vi "信号光谱9 -grating.vi"() -> ()   [LabVIEW 2018]
uses:
  <vilib>/Utility/NIReport.llb/Report Type.ctl
  <vilib>/Instr/_visa.llb/VISA Configure Serial Port (Instr).vi
  <vilib>/addons/_office/excel.llb/Excel Get Data ([str]).vi
  <vilib>/Utility/file.llb/Write Delimited Spreadsheet (DBL).vi
  <vilib>/Utility/NIReport.llb/NI_report.lvclass
  <vilib>/Analysis/NI_AALBase.lvlib
  <vilib>/Utility/NIReport.llb/NI_ReportGenerationCore.lvlib
  <vilib>/addons/_office/NI_ReportGenerationToolkit.lvlib
  <vilib>/Utility/NIReport.llb/Excel/NI_Excel.lvclass
panel:
  in  "C=w-w0":dbl=1800.0 format="%#_13g"
  in  "Target WL 2":dbl=552.444
  in  "判断角度上限":dbl=4.0 format="%#_13g"
  in  "判断角度下限":dbl=1.0 format="%#_13g"
  in  "角度倍乘系数":dbl=1.5
  out "Δw2>C":bool=TRUE
  out "Δw1>C":bool=TRUE
  out "θi":dbl
  in  "上升下降沿/s":dbl format="%.2p"
  in  "延时/s":dbl format="%.2p"
  in  "占空比/%":dbl=3.0 format="%.2p"
  in  "高电平/V":dbl=4.0 format="%.2p"
  in  "频率/Hz":dbl=6000.0 format="%.3p"
  in  "低电平/V":dbl min=0.0 max=5.0 format="%.2p"
  in  "Enable":bool
  in  "上升下降沿":i32(ring)=1 items=["上升沿", "下降沿"]
  in  "输出信号波形":u16(ring) items=["Pulse"]
  out "Output":bool
  in  "VISA 信号发生器":refnum<visa-resource-name>="USB0::0x1AB1::0x0641::DG4E192200870::INSTR"
  out "Output 2":bool
  in  "Enable 2":bool
  in  "上升下降沿/s 2":dbl format="%.2p"
  in  "延时/s 2":dbl format="%.2p"
  in  "占空比/% 2":dbl=3.0 format="%.2p"
  in  "高电平/V 2":dbl=0.002 format="%.2p"
  in  "频率/Hz 2":dbl=6000.0 format="%.3p"
  in  "低电平/V 2":dbl min=0.0 max=5.0 format="%.2p"
  in  "上升下降沿 2":i32(ring)=1 items=["上升沿", "下降沿"]
  in  "输出信号波形 2":u16(ring) items=["Pulse"]
  in  "终止测量":bool
  in  "测量次数":i32=1
  out "angle":dbl
  out "图片地址":string
  in  "开光时间/ms":u32=50
  out "最终存储路径 2":path
  out "照明光error out":errorcluster
  in  "照明光":bool
  in  "stop bits (10: 1 bit)":u16(ring)=10 items=["1.0"=10, "1.5"=15, "2.0"=20]
  in  "parity (0:none)":enum16{"None", "Odd", "Even", "Mark", "Space"}(ring)
  in  "data bits (8)":u16=8 min=5 max=8 step=1
  in  "baud rate":u32=9600 caption="baud rate (115200)" min=9600 max=115200
  in  "照明光VISA":refnum<visa-resource-name>="COM5"
  out "正在测量":bool
  out "最终存储路径":path
  in  "停止程序":bool
  out "configure error out":errorcluster
  in  "设置参数":bool
  out "output control error  4":errorcluster
  in  "低电平持续输出":bool
  out "output control error  5":errorcluster
  out "output control error":errorcluster
  in  "开始测量":bool
  in  "channel输出口":i32(ring) items=["Channel 1", "Channel 2"]
  out "output control error":errorcluster
  out "Spectrum":cluster{"Y":dbl[], "Y":dbl[]}[](graph)
  out "波长范围":dbl[](array[numeric])
  in  "?":enum32{"IHR 550", "CCD"}(tab)
  in  "Move To\nTarget Positions":bool
  out "Current UniqueID":string="Mono4"
  in  "Mono ID":string(combo)="Mono1"
  in  "Connect":bool
  out "Initialized JY":bool=TRUE
  in  "Force\nInitialization":bool
  in  "Target Grating":string(combo)="2"
  out "Current Description":string="1" caption="Description"
  out "Grating Index":i32=1
  out "Current Grating":dbl=1200.0
  out "Units":string="nm"
  out "Current WL":dbl=897.9988
  out "Exit Mirror\nPosition":i32(ring)=2 items=["EntranceMirror", "ExitMirror", "Front", "Side"]
  out "Entrance Mirror\nPosition":i32(ring)=2 items=["EntranceMirror", "ExitMirror", "Front", "Side"]
  out "Units 2":string="mm"
  out "Front Entrance":dbl
  in  "Target WL":dbl=517.603
  in  "Exit Mirror":u16(ring)=3 caption="Target Position Exit Mirror" items=["Front"=2, "Side"=3]
  in  "Entrance Mirror":u16(ring)=2 caption="Target Position\nEntrance Mirror" items=["Front"=2, "Side"=3]
  in  "Target\nFront Entrance":dbl=2.0
  in  "操作":bool
  in  "Commande tab":T1(tab)
  in  "Area Number to Display":i32
  in  "Reformat":bool
  in  "GAIN":u16(ring)=2 caption="Device Name" items=["High Light", "Best Dynamic Range", "High Sensitivity"]
  in  "ADC":u16(ring) caption="Device Name" items=["20 kHz       ", " 1 MHz       ", " 1 MHz Ultra "]
  in  "Number of Areas :":u16=1 min=1 step=1
  in  "Integration time (ms) :":i16=1000
  out "Uniques ID":u16(ring) items=["CCD1", "CCD2"]
  in  "Device Name":u16(ring) items=["Synapse CCD (Lateral)", "Synapse_IGA (Axial)"]
  in  "Signal type :":enum16{"TTL Rising Edge", "TTL Falling Edge"}(ring)=enum."TTL Falling Edge"
  in  "Trigger Type :":u16(ring) items=["On Start"=1, "Per Acquisition"=2]
  in  "trigSigTypeString":string
  in  "trigEventString":string
  in  "Enable InputTriggers :":bool
  in  "Number of Cleans":i32=1
  in  "MultiAcqShutterMode":i32(ring)=3 items=["Open For All Spectra"=1, "Open for Each Spectrum"=3]
  in  "Accumulations:":u16=10 min=1 step=1
  in  "Multi Accumulation mode:":bool
  out "Y Pixels:":i32=256
  out "DataSize":i32=1024
  out "X Pixels:":i32=1024
  out "Firmware\nVersion":string="V1.20 CCD_4000"
  out "initialized ?":bool=TRUE
  in  "Continuous":bool
  in  "CCD Busy":bool
  out "indicator":string="Ready !"
  in  "initialize":bool
  in  "ShutterOpen":bool=TRUE caption="Shutter enable"
  in  "Acquire":bool
  in  "Temperature":bool
  in  "Setup":bool
  out "Acq Time(ms)":u32=3401
  in  "Save Backlight":bool
  in  "cut backlight":bool
  out "backlight":bool=TRUE
  in  "是否保存":bool
  in  "Close":bool=TRUE
  out "JYCCDLib.IJYCCDReqd":refnum<k7>
  out "areas :":i32[][](array[numeric])=[[1], [1], [1], [1024], [256], [1], [256]]
  in  "Constante de condition\n(Voir l'aide contextuelle)":bool
  out "temp graph":dbl(graph)=-134.538067
  out "ADC Number":i32[](array[numeric])=[0, 1, 2, 3, 4]
  out "Gain Number":i32[](array[numeric])=[10, 11, 12, 13, 8, 2]
  out "trigAddress":i32
  out "Data":i32[][](graph)
  out "error out":errorcluster
  out "Gratings":dbl[](array[numeric])=[1200.0, 300.0]
  out "Backlight":i32[][](graph)
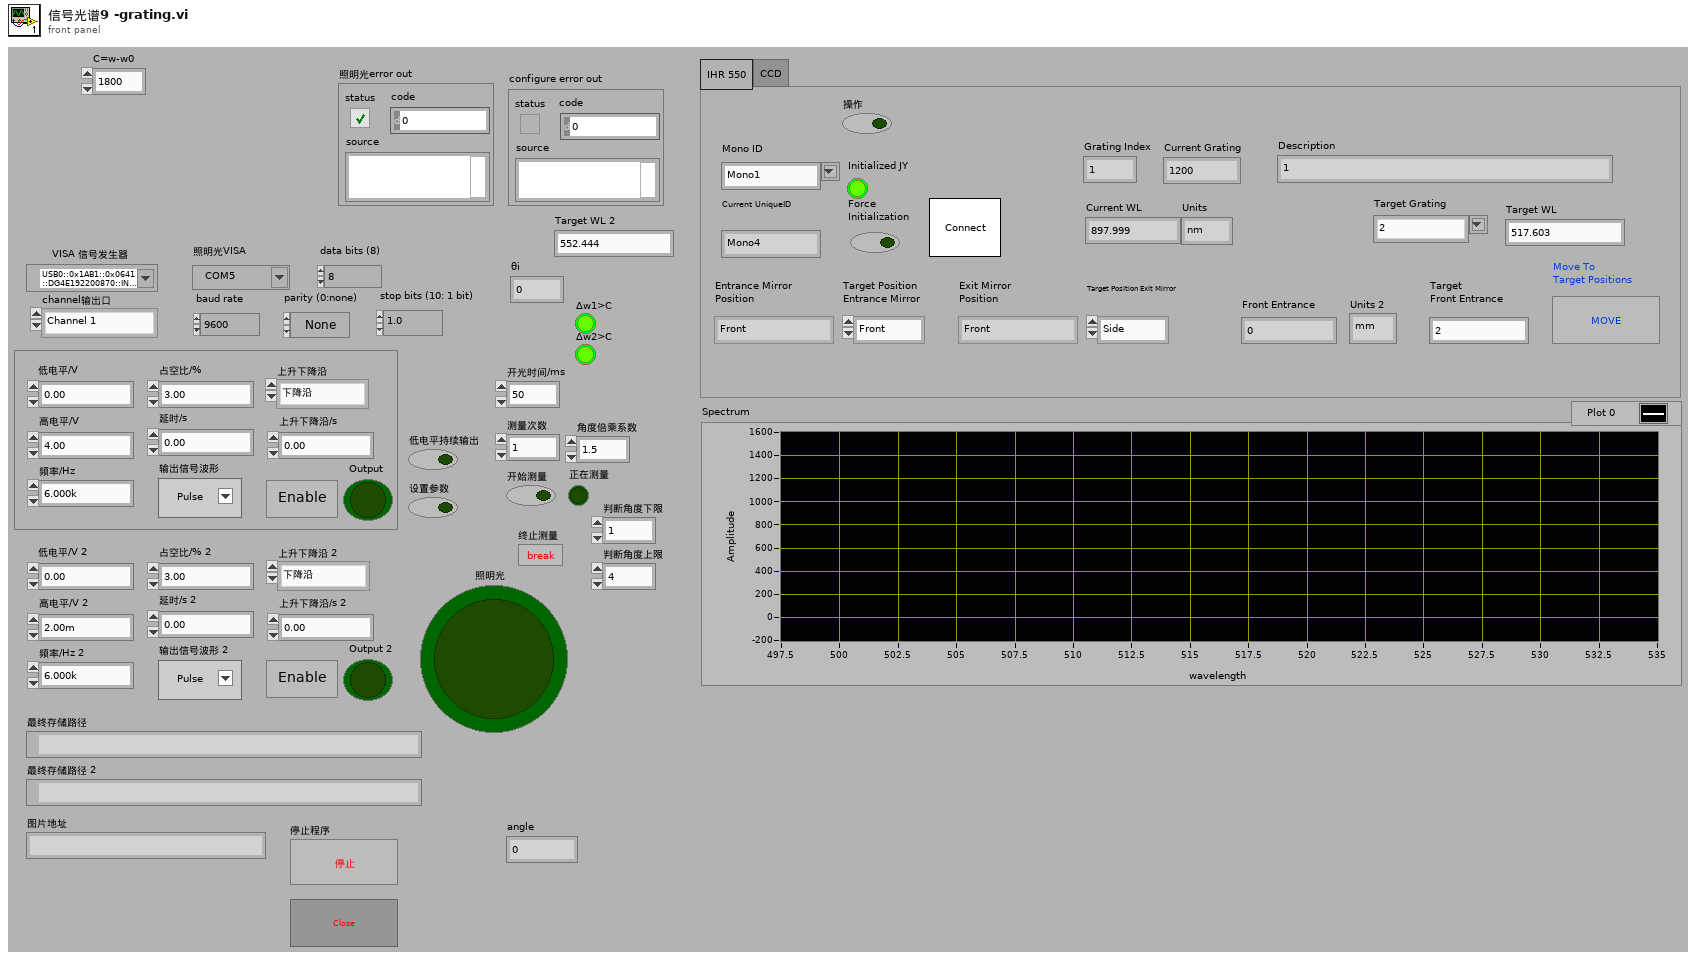
[diagram p1: front panel]
types:
  T1 = enum32{"Settings", "Trigger In", "Multi-Accu.", "Infos"}
  T2 = enum8{"Enabled", "Disabled", "Disabled and Grayed Out"}
  T3 = enum16{"maximized", "minimized", "normal", "no change"}
  T4 = typedef "NI_ReportGenerationCore.lvlib/Report Type.ctl" = enum16{"HTML", "Word", "Excel"}
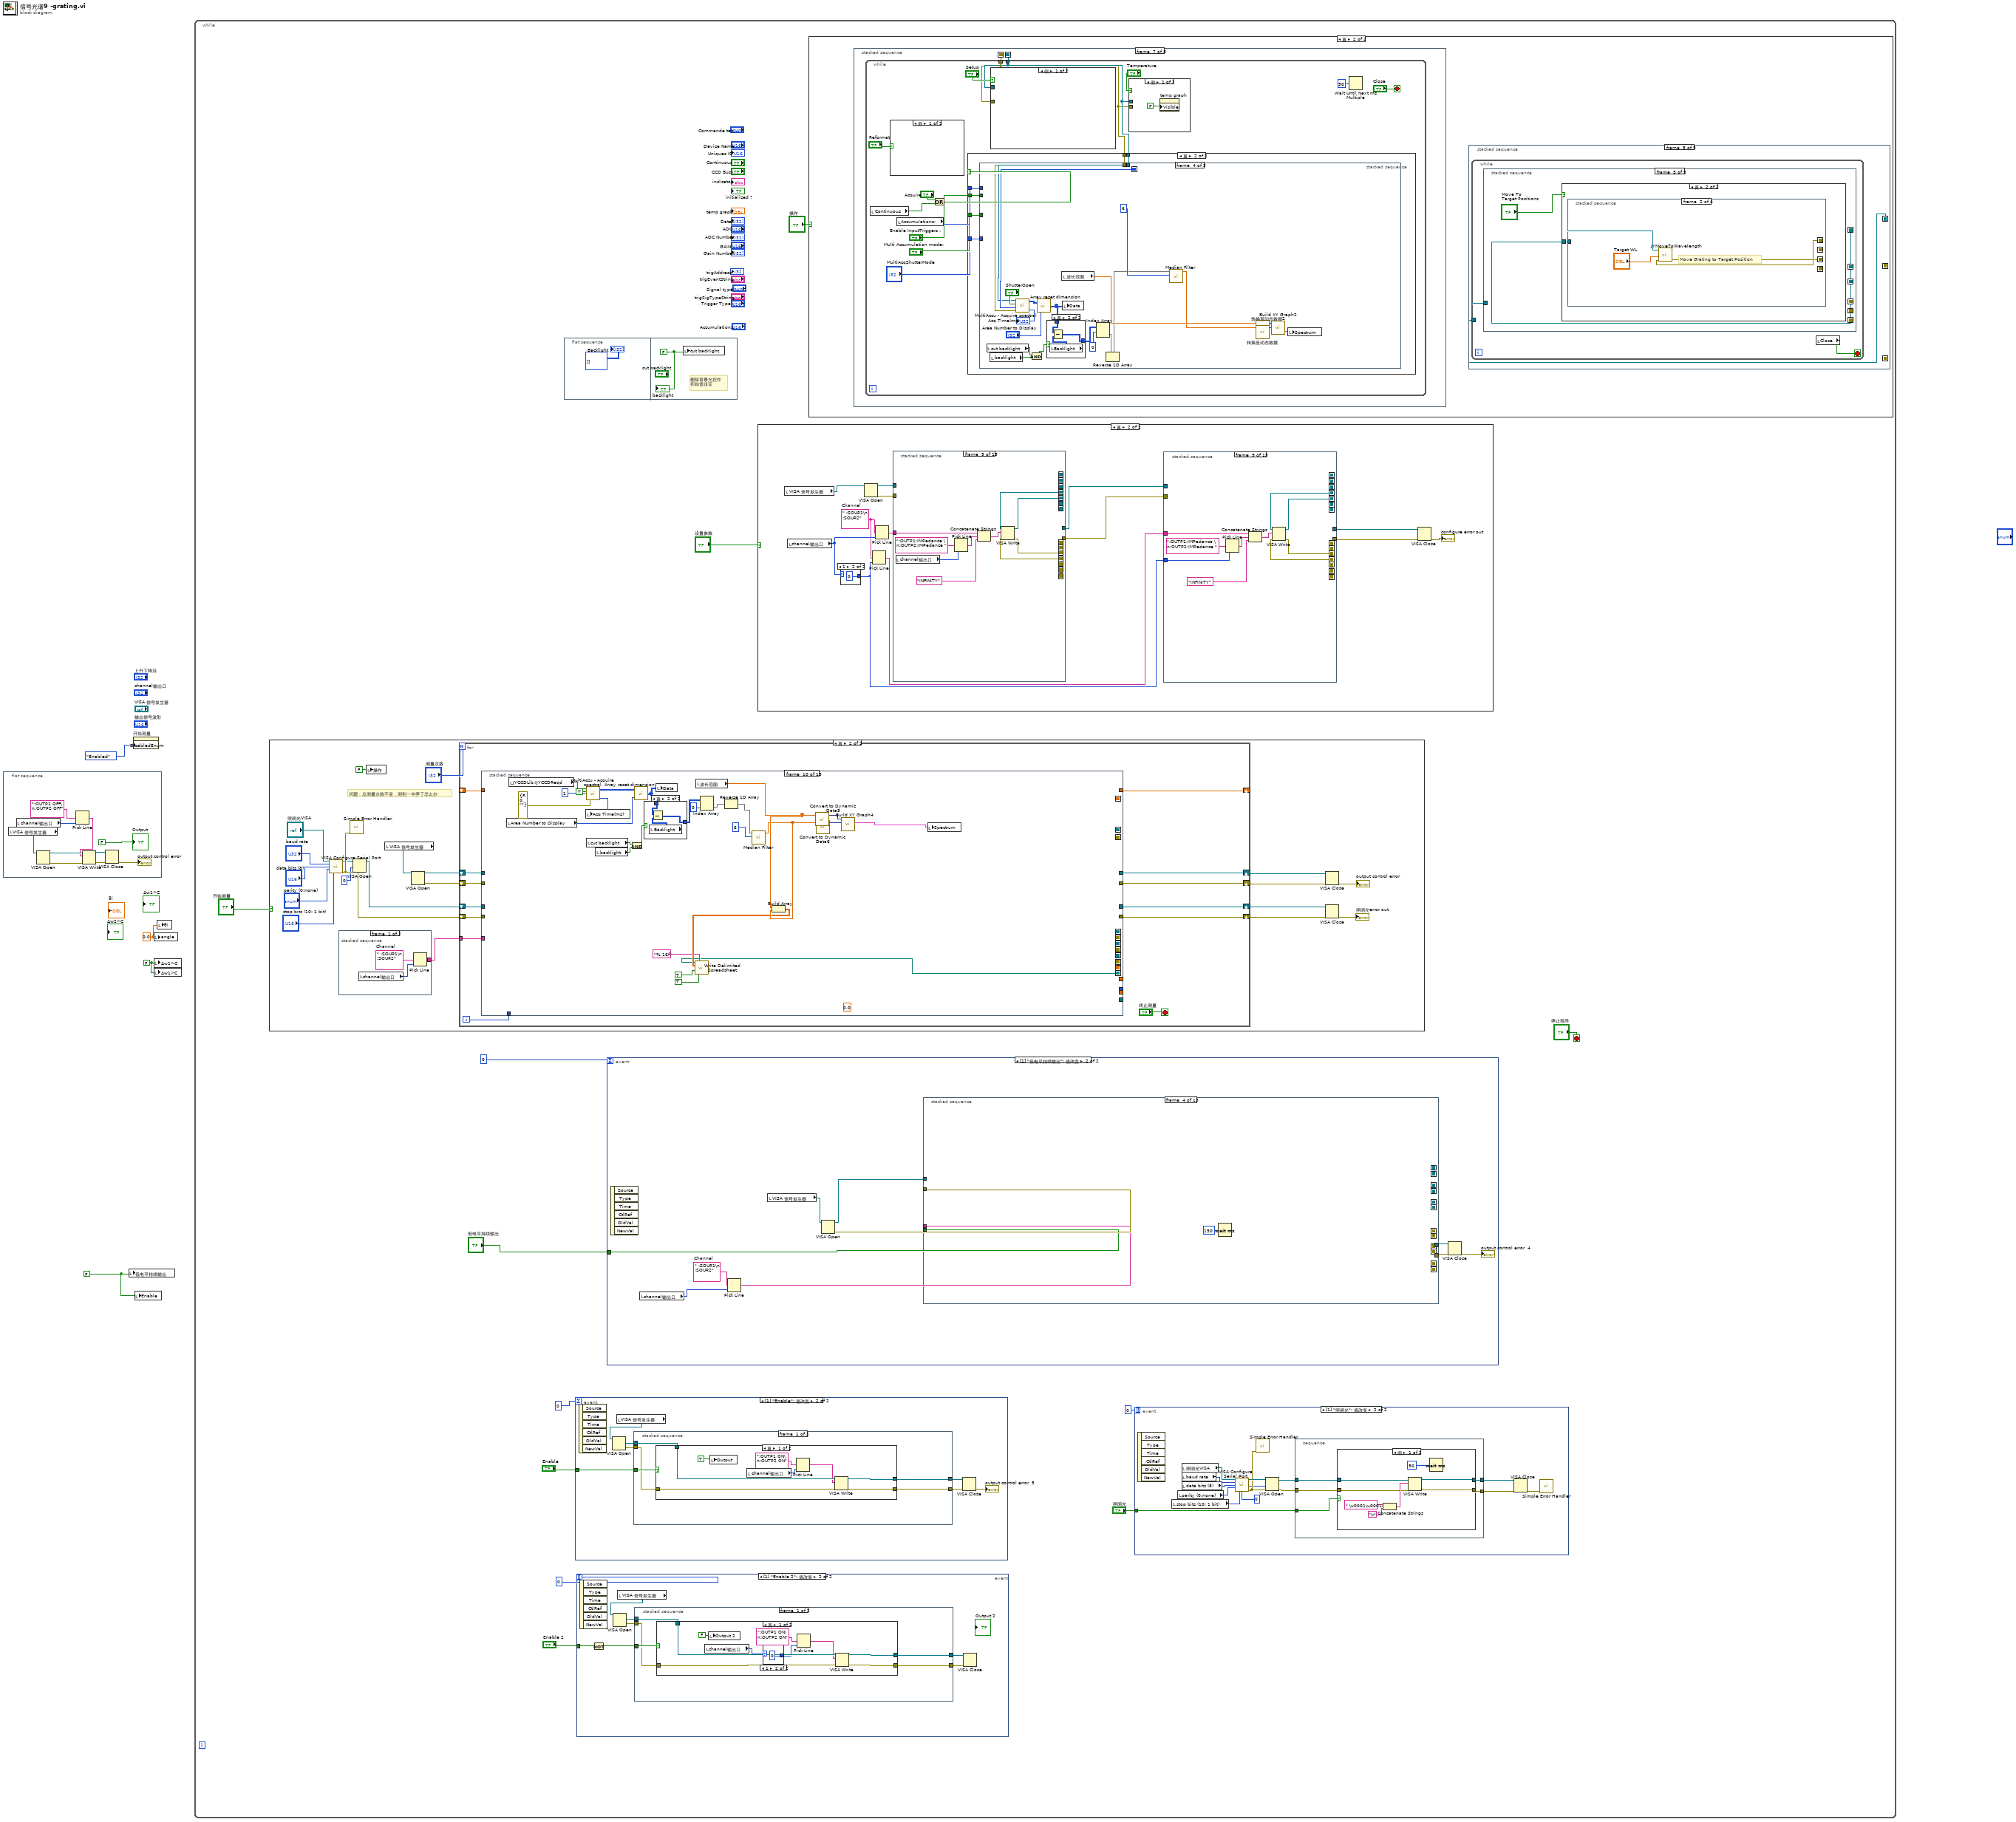
[diagram p0: block diagram]
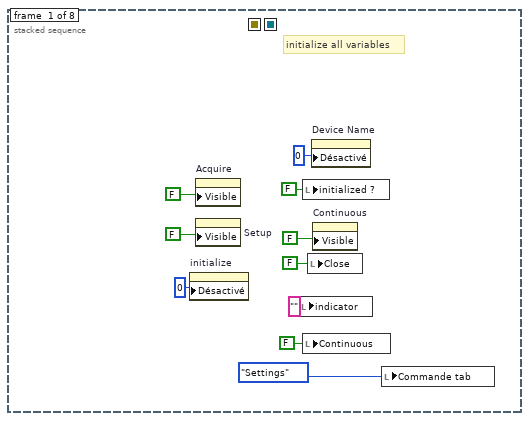
[diagram p3: hidden frame]
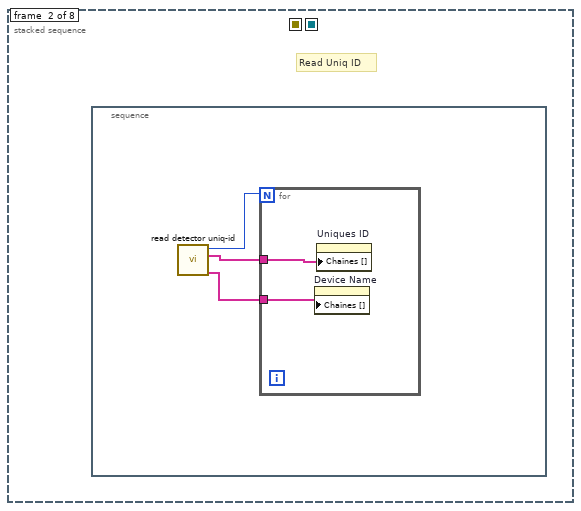
[diagram p4: hidden frame]
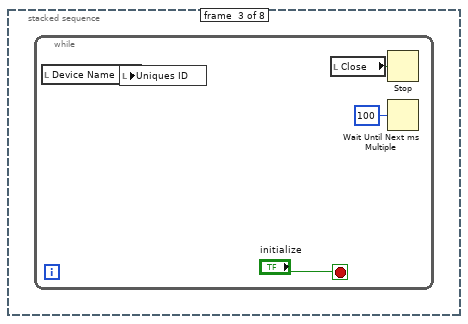
[diagram p5: hidden frame]
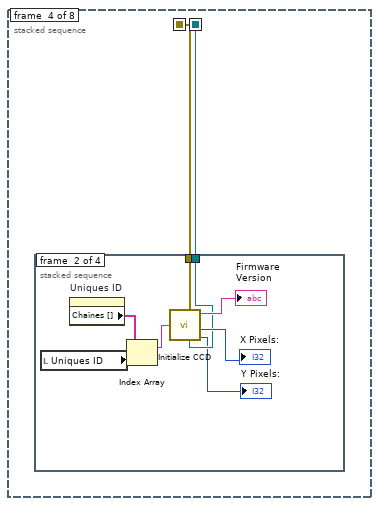
[diagram p6: hidden frame]
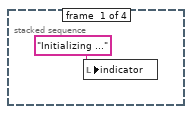
[diagram p7: hidden frame]
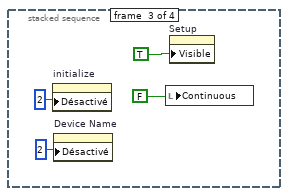
[diagram p8: hidden frame]
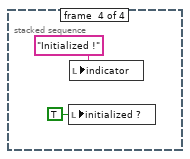
[diagram p9: hidden frame]
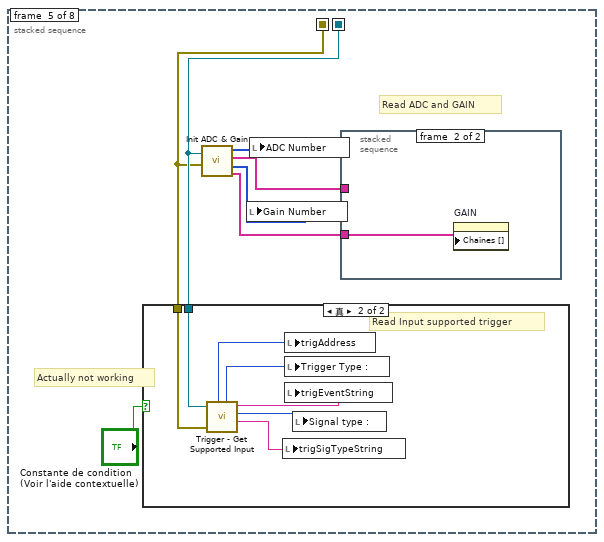
[diagram p10: hidden frame]
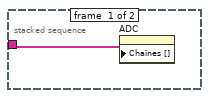
[diagram p12: hidden frame]
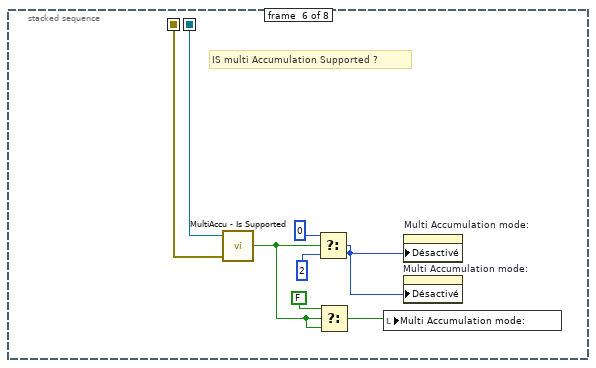
[diagram p13: hidden frame]
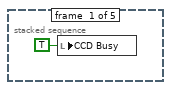
[diagram p15: hidden frame]
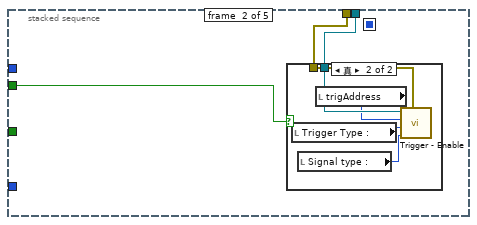
[diagram p16: hidden frame]
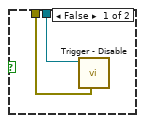
[diagram p17: hidden frame]
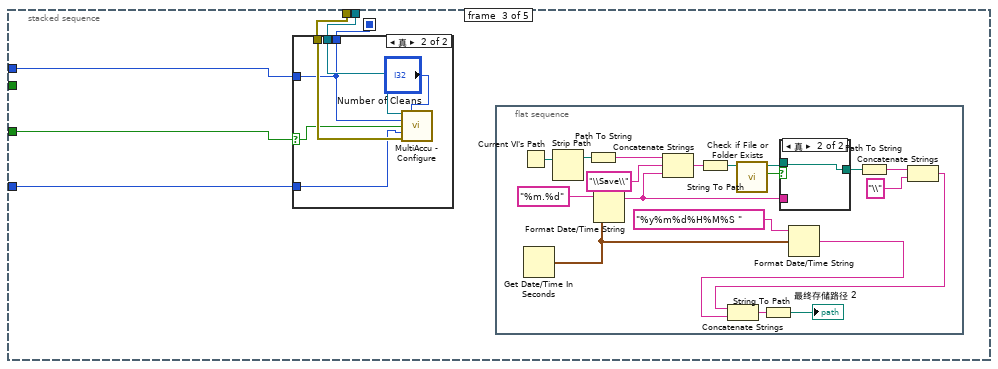
[diagram p18: hidden frame]
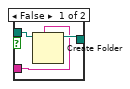
[diagram p19: hidden frame]
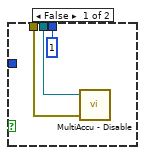
[diagram p20: hidden frame]
diagram:
  w1 = FALSE ("Δw1>C")
  w2 = 0.0 ("angle")
  w3 = FALSE
  n1 = flat-sequence {
    frame #0 {
      n2 = local read "VISA 信号发生器"() -> (w8:refnum<visa-resource-name>)
      n3 = local read "channel输出口"() -> (w6:i32)
      n4 = VISA Open(VISA resource name=w8) -> (VISA resource name=w14:refnum<visa-resource-name>, error out=w13:errorcluster)  [unwired: 4 in]
      n5 = Pick Line(multi-line string=":OUTP1 OFF\n:OUTP2 OFF" ("write buffer"), line index=w6) -> (output string=w5:string)  [unwired: 1 in]
      n6 = VISA Write(VISA resource name=w14, write buffer=w5, error in (no error)=w13) -> (VISA resource name out=w11:refnum<visa-resource-name>, error out=w10:errorcluster)  [unwired: 1 out]
      n7 = VISA Close(VISA resource name=w11, error in (no error)=w10) -> (error out=→"output control error":errorcluster)
      "Output" <- FALSE ("布尔")
    }
  }
  n8 = local write "低电平持续输出"(w3) -> ()
  n9 = property on="开始测量" class="Bool"("DisabledEnum"=T2."Enabled" ("禁用")) -> ()  [unwired: 2 in, 2 out]
  n10 = local write "Enable"(w3) -> ()
  n11 = local write "angle"(w2) -> ()
  n12 = local write "Δw1>C"(w1) -> ()
  n13 = local write "Δw1>C"(w1) -> ()
  n14 = local write "θi"(w2) -> ()
  n15 = while {
    stop <- "停止程序" stop-if-true
    n16 = case shown="真" "开始测量" {
      frame False {
      }
      frame True {
        # "问题：总测量次数不变，测到一半停了怎么办"
        n17 = call-poly "VISA Configure Serial Port"("VISA resource name"="照明光VISA", "baud rate (9600)"="baud rate", "data bits (8)"="data bits (8)", "parity (0:none)"="parity (0:none)", "stop bits (10: 1 bit)"="stop bits (10: 1 bit)") -> ("VISA resource name out"=w411:refnum<visa-resource-name>, "error out"=w412:errorcluster)  [unwired: 9 in]
        n18 = stacked-sequence {
          tunnel: [w421 _] -> w415
          frame #0 {
            w422 = " :SOUR1\n :SOUR2"  # Channel
            n19 = local read "channel输出口"() -> (w423:i32)
            n20 = Pick Line(multi-line string=w422, line index=w423) -> (output string=w421:string)  [unwired: 1 in]
          }
          frame #1 {
            w424 = FALSE ("Δw1>C")
            n21 = local write "Δw1>C"(w424) -> ()
            n22 = local write "Δw2>C"(w424) -> ()
          }
        }
        n23 = call <vilib>:"Simple Error Handler.vi"("error in (no error)"=w412) -> ()  [unwired: 4 in, 5 out]
        n24 = VISA Open(access mode=0, error in (no error)=w412, VISA resource name=w411) -> (VISA resource name=w404:refnum<visa-resource-name>, error out=w403:errorcluster)  [unwired: 2 in]
        n25 = local write "操作"(FALSE ("操作")) -> ()
        n26 = local read "VISA 信号发生器"() -> (w420:refnum<visa-resource-name>)
        n27 = VISA Open(VISA resource name=w420) -> (VISA resource name=w419:refnum<visa-resource-name>, error out=w418:errorcluster)  [unwired: 4 in]
        n28 = for {
          N: "测量次数" -> [_]
          tunnel: w415 -> [w435]
          shift-right: [w431] -> w414
          shift-left: w419 -> [w437]
          shift-right: [w430] -> w413
          shift-left: w418 -> [w436]
          shift-right: [w429] -> w417
          shift-left: w404 -> [w434]
          shift-right: [w428] -> w416
          shift-left: w403 -> [w433]
          shift-right: [w427] -> _
          shift-left: _ -> [w426]
          i -> [w425]
          stop <- "终止测量" stop-if-true
          n29 = stacked-sequence {
            seq-local: [w444 _ _ _ _ _ _ _ _ _ _ _ _ _ _] -> [_ w464 _ _ _ _ _ _ _ _ _ _ _ _ _]
            seq-local: [w443 _ _ _ _ _ _ _ _ _ _ _ _ _ _] -> [_ w463 _ _ _ _ _ _ _ _ _ _ _ _ _]
            seq-local: [_ _ _ _ _ w549 _ _ _ _ _ _ _ _ _] -> [_ _ _ _ _ _ _ _ _ _ _ w677 _ _ _]
            seq-local: [_ _ _ _ _ w548 _ _ _ _ _ _ _ _ _] -> [_ _ _ _ _ _ _ _ _ _ _ w680 _ _ _]
            seq-local: [_ w462 _ _ _ _ _ _ _ _ _ _ _ _ _] -> [_ _ _ _ w535 _ _ _ _ _ _ _ _ _ _]
            seq-local: [_ w461 _ _ _ _ _ _ _ _ _ _ _ _ _] -> [_ _ _ _ w534 _ _ _ _ _ _ _ _ _ _]
            seq-local: [_ _ _ _ w533 _ _ _ _ _ _ _ _ _ _] -> [_ _ _ _ _ _ _ _ _ _ w663 _ _ _ _]
            seq-local: [_ _ _ _ w532 _ _ _ _ _ _ _ _ _ _] -> [_ _ _ _ _ _ _ _ _ _ w662 _ _ _ _]
            seq-local: [_ _ w473 _ _ _ _ _ _ _ _ _ _ _ _] -> [_ _ _ _ _ _ _ _ _ _ _ _ _ w688 _]
            seq-local: [w438 _ _ _ _ _ _ _ _ _ _ _ _ _ _] -> [_ _ _ _ _ _ _ _ _ _ _ _ _ _ _]
            seq-local: [_ _ _ _ _ _ _ w568 _ _ _ _ _ _ _] -> [_ _ _ _ _ _ _ _ _ w630 _ _ _ _ _]
            tunnel: w437 -> [w446 _ _ _ _ _ _ _ _ _ _ _ _ _ _]
            tunnel: w436 -> [w445 _ _ _ _ _ _ _ _ _ _ _ _ _ _]
            tunnel: [_ _ _ _ _ _ _ _ _ _ w661 _ _ _ _] -> w431
            tunnel: [_ _ _ _ _ _ _ _ _ _ w660 _ _ _ _] -> w430
            tunnel: w435 -> [_ _ _ _ _ _ _ _ _ _ _ _ _ _ _]
            tunnel: w434 -> [_ _ _ _ _ w552 _ _ _ _ _ _ _ _ _]
            tunnel: w433 -> [_ _ _ _ _ w551 _ _ _ _ _ _ _ _ _]
            tunnel: [_ _ _ _ _ _ _ _ _ _ _ w679 _ _ _] -> w429
            tunnel: [_ _ _ _ _ _ _ _ _ _ _ w678 _ _ _] -> w428
            tunnel: [_ _ w473 _ _ _ _ _ _ _ _ _ _ _ _] -> _
            tunnel: [_ _ _ w507 _ _ _ _ _ _ _ _ _ _ _] -> _
            tunnel: [w438 _ _ _ _ _ _ _ _ _ _ _ _ _ _] -> _
            tunnel: [_ _ w473 _ _ _ _ _ _ _ _ _ _ _ _] -> w427
            tunnel: w426 -> [_ _ _ _ _ _ _ _ _ _ _ _ _ w687 _]
            tunnel: w425 -> [_ _ _ _ _ _ _ _ _ _ _ _ _ w685 _]
            tunnel: [_ _ _ w506 _ _ _ _ _ _ _ _ _ _ _] -> _
            frame #0 {
              n30 = Wait Until Next ms Multiple(millisecond multiple=u32 1 ("毫秒倍数")) -> ()  [unwired: 1 out]
              n31 = flat-sequence {
                tunnel: w446 -> [w460]
                tunnel: w445 -> [w459]
                tunnel: [w454] -> w444
                tunnel: [w453] -> w443
                frame #0 {
                  n32 = local read "channel输出口"() -> (w456:i32)
                  n33 = local write "Output"(TRUE ("布尔")) -> ()
                  n34 = Pick Line(multi-line string=":OUTP1 ON\n:OUTP2 ON" ("write buffer"), line index=w456) -> (output string=w455:string)  [unwired: 1 in]
                  n35 = VISA Write(VISA resource name=w460, write buffer=w455, error in (no error)=w459) -> (VISA resource name out=w454:refnum<visa-resource-name>, error out=w453:errorcluster)  [unwired: 1 out]
                }
              }
              n36 = local read "Δw1>C"() -> (w440:bool)
              n37 = local read "Δw2>C"() -> (w441:bool)
              n38 = And(x=w440, y=w441) -> (x .and. y?=w439:bool)
              n39 = case shown="假" w439 {
                tunnel: [w449 w450] -> w438
                tunnel: "开光时间/ms" -> [w449 w452]
                frame False {
                }
                frame True {
                  n40 = Divide(x=w452, y=u32 4) -> (x/y=w450:dbl)
                }
              }
              n41 = Wait (ms)(milliseconds to wait=w438) -> ()  [unwired: 1 out]
              "正在测量" <- TRUE
            }
            frame #1 {
              n42 = flat-sequence {
                tunnel: w464 -> [w472]
                tunnel: w463 -> [w471]
                tunnel: [w466] -> w462
                tunnel: [w465] -> w461
                frame #0 {
                  n43 = local read "channel输出口"() -> (w468:i32)
                  n44 = local write "Output"(FALSE ("布尔")) -> ()
                  n45 = Pick Line(multi-line string=":OUTP1 OFF\n:OUTP2 OFF" ("write buffer"), line index=w468) -> (output string=w467:string)  [unwired: 1 in]
                  n46 = VISA Write(VISA resource name=w472, write buffer=w467, error in (no error)=w471) -> (VISA resource name out=w466:refnum<visa-resource-name>, error out=w465:errorcluster)  [unwired: 1 out]
                }
              }
            }
            frame #2 {
              n47 = stacked-sequence {
                seq-local: [_ w487 _ _] -> [_ _ w488 w497]
                tunnel: [_ _ _ w496] -> w473
                frame #0 {
                  n48 = Get Date/Time In Seconds() -> (seconds since 1Jan1904=w483:timestamp)
                  n49 = Get Date/Time String(date format (0)=enum16{"short", "long", "abbreviated"}."abbreviated" ("日期格式(0)"), seconds (now)=w483, want seconds? (F)=TRUE ("需要秒？(F)")) -> (date string=w486:string, time string=w484:string)
                  n50 = Search and Replace String(replace all?=TRUE ("替换全部？(F)"), input string=w484, search string=":" ("搜索字符串"), replace string="-" ("替换字符串(\"\")")) -> (result string=w485:string)  [unwired: 4 in, 3 out]
                  n51 = Concatenate Strings("D:\\desktop\\train\\photo\\", w486, w485, "光谱" ("字符串"), ".jpg" ("字符串")) -> (→"图片地址":string)
                }
                frame #1 {
                  # "SaveImage"
                  n52 = local read "图片地址"() -> (w487:string)
                }
                frame #2 {
                  n53 = Open Python Session(python version="3.9" ("Python version")) -> (session out=w495:refnum<k35>, error out=w493:errorcluster)  [unwired: 2 in]
                  n54 = node(w495, path "D:/desktop/train/model/main.py" ("module path"), "screenshot" ("function name"), w493, w488) -> (w494:refnum<k35>, w492:errorcluster)  [unwired: 3 in, 2 out]
                  n55 = Close Python Session(session in=w494, error in=w492) -> ()  [unwired: 1 out]
                }
                frame #3 {
                  n56 = Open Python Session(python version="3.9" ("Python version")) -> (session out=w504:refnum<k35>, error out=w502:errorcluster)  [unwired: 2 in]
                  n57 = node(w504, path "D:/desktop/train/newpro.py" ("module path"), "fun" ("function name"), w502, 0.0, w497) -> (w503:refnum<k35>, w501:errorcluster, w496:dbl)  [unwired: 1 in, 2 out]
                  "angle" <- w496
                  n58 = Close Python Session(session in=w503, error in=w501) -> ()  [unwired: 1 out]
                }
              }
            }
            frame #3 {
              n59 = Current VI's Path() -> (path=w516:path)
              n60 = Get Date/Time In Seconds() -> (seconds since 1Jan1904=w509:timestamp)
              n61 = Strip Path(path=w516) -> (stripped path=w517:path)  [unwired: 1 out]
              n62 = Path To String(path=w517) -> (string=w518:string)
              n63 = Format Date/Time String(time format string (%c)="%m-%d" ("时间格式字符串(%c)"), seconds (now)=w509) -> (date/time string=w524:string)  [unwired: 1 in]
              n64 = Concatenate Strings(w518, "\\Save\\" ("字符串"), w524) -> (w519:string)
              n65 = String To Path(string=w519) -> (path=w520:path)
              n66 = call <vilib>:"Check if File or Folder Exists.vi"("path"=w520) -> ("file or folder exists?"=w521:bool, "dup path"=w523:path)  [unwired: 8 in, 1 out]
              n67 = case shown="真" w521 {
                tunnel: [w530 w531] -> w522
                tunnel: w523 -> [w529 w531]
                tunnel: w524 -> [w528 _]
                frame False {
                  n68 = Create Folder(prompt (Create Folder)=w528, path (use dialog)=w529) -> (created path=w530:path)  [unwired: 1 in, 2 out]
                }
                frame True {
                }
              }
              n69 = Format Date/Time String(time format string (%c)="%y%m%d%H%M%S" ("时间格式字符串(%c)"), seconds (now)=w509) -> (date/time string=w527:string)  [unwired: 1 in]
              n70 = Path To String(path=w522) -> (string=w525:string)
              n71 = Concatenate Strings(w525, "\\" ("字符串")) -> (w526:string)
              n72 = Format Date/Time String(time format string (%c)="%H%M%S" ("时间格式字符串(%c)"), seconds (now)=w509) -> (date/time string=w508:string)  [unwired: 1 in]
              n73 = Concatenate Strings(w526, w527) -> (w515:string)
              n74 = String To Path(string=w515) -> (path=w506:path)
              "最终存储路径" <- w506
              n75 = Decimal String To Number(string=w508) -> (number=w507:i32)  [unwired: 2 in, 1 out]
            }
            frame #4 {
              n76 = flat-sequence {
                tunnel: w535 -> [w544]
                tunnel: w534 -> [w543]
                tunnel: [w539] -> w533
                tunnel: [w538] -> w532
                frame #0 {
                  n77 = local read "channel输出口"() -> (w537:i32)
                  n78 = case shown="1" w537 {
                    tunnel: [1 0] -> w536
                    frame 0, Default {
                    }
                    frame 1 {
                    }
                  }
                  n79 = local write "Output 2"(FALSE ("布尔")) -> ()
                  n80 = Pick Line(multi-line string=":OUTP1 OFF\n:OUTP2 OFF" ("write buffer"), line index=w536) -> (output string=w540:string)  [unwired: 1 in]
                  n81 = VISA Write(VISA resource name=w544, write buffer=w540, error in (no error)=w543) -> (VISA resource name out=w539:refnum<visa-resource-name>, error out=w538:errorcluster)  [unwired: 1 out]
                }
              }
            }
            frame #5 {
              w547 = " \u0001\u0001¢"  # Channel
              n82 = Wait (ms)(milliseconds to wait=1200) -> ()  [unwired: 1 out]
              n83 = Concatenate Strings(w547, "\r") -> (w553:string)
              n84 = local write "照明光"(FALSE ("照明光")) -> ()
              n85 = VISA Write(VISA resource name=w552, write buffer=w553, error in (no error)=w551) -> (VISA resource name out=w549:refnum<visa-resource-name>, error out=w548:errorcluster)  [unwired: 1 out]
            }
            frame #6 {
              n86 = flat-sequence {
                frame #0 {
                  n87 = call <vilib>:"Create Report.vi"("window state (normal)"=T3."no change", "report type"=Report_Type."Excel", "template (empty)"=path "D:/desktop/train/TEST1/Save/516中心波长.xlsx") -> ("report out"=w562:refnum<class "NI_report.lvclass">, "error out"=w561:errorcluster)  [unwired: 11 in]
                  n88 = call-poly <vilib>:"Excel Get Data.vi"("report in"=w562, "data type"=string[][] [], "error in (no error)"=w561) -> ("report out"=w557:refnum<class "NI_report.lvclass">, "data"=w565:string[][], "error out"=w556:errorcluster)  [unwired: 10 in]
                  n89 = call-dynamic "Dispose Report.vi"("report in"=w557, "error in (no error)"=w556) -> ()  [unwired: 13 in, 1 out]
                  n90 = Index Array(array=w565, index (col)=0 ("禁用的索引 (列)")) -> (element=w567:string[])  [unwired: 1 in]
                  n91 = Fract/Exp String To Number(string=w567) -> (number=→"波长范围":dbl[])  [unwired: 3 in, 1 out]
                }
              }
            }
            frame #7 {
              (unwired) 0.0 ("元素")
              n92 = local read "Area Number to Display"() -> (w584:i32)
              n93 = local read "JYCCDLib.IJYCCDReqd"() -> (w580:refnum<k7>)
              n94 = Get Date/Time In Seconds() -> (seconds since 1Jan1904=w593:timestamp)
              n95 = local read "最终存储路径"() -> (w606:path)
              n96 = Get Date/Time String(date format (0)=enum16{"short", "long", "abbreviated"}."abbreviated" ("日期格式(0)"), seconds (now)=w593, want seconds? (F)=TRUE ("需要秒？(F)")) -> (date string=w601:string, time string=w596:string)
              n97 = call "MultiAccu - Acquire spectral.vi"("error in"=errorcluster {"status"=FALSE, "code"=0, "source"=""}, "Accumulations:"=u16 1, "ShutterOpen"=TRUE, "JYCCDLib.IJYCCDReqd"=w580) -> ("Acq Time(ms)"=w586:u32, "Array Out"=w585:i32[][][])  [unwired: 1 out]
              n98 = local write "Acq Time(ms)"(w586) -> ()
              n99 = local read "cut backlight"() -> (w575:bool)
              n100 = local read "backlight"() -> (w573:bool)
              n101 = Search and Replace String(replace all?=TRUE ("替换全部？(F)"), input string=w596, search string=":" ("搜索字符串"), replace string="-" ("替换字符串(\"\")")) -> (result string=w600:string)  [unwired: 4 in, 3 out]
              n102 = Path To String(path=w606) -> (string=w590:string)
              n103 = And(x=w575, y=w573) -> (x .and. y?=w574:bool)
              n104 = call "Array reset dimension.vi"("Area Number"=w584, "Array In"=w585) -> ("Array Out"=w577:i32[][])
              n105 = Concatenate Strings(w590, w601, w600, "光谱" ("字符串"), ".xls" ("字符串")) -> (w605:string)
              n106 = case shown="真" w574 {
                tunnel: [w608 w610] -> w576
                tunnel: w577 -> [w608 w609]
                frame False {
                }
                frame True {
                  n107 = local read "Backlight"() -> (w611:i32[][])
                  n108 = Subtract(x=w609, y=w611) -> (x-y=w610:i32[][])
                }
              }
              n109 = String To Path(string=w605) -> (path=w568:path)
              n110 = local write "Data"(w577) -> ()
              n111 = local read "波长范围"() -> (w571:dbl[])
              n112 = Index Array(array=w576, index (row)=0 ("索引 (行)")) -> (element=w607:i32[])  [unwired: 1 in]
              n113 = Reverse 1D Array(array=w607) -> (reversed array=w572:i32[])
              n114 = call <vilib>:"Median Filter.vi"("left rank"=6, "X"=w572) -> ("Filtered X"=w570:dbl[])  [unwired: 8 in, 1 out]
              n115 = Build Array(w571, w570) -> (w569:dbl[][])
              n116 = call-poly <vilib>:"Write Delimited Spreadsheet.vi"("file path (dialog if empty)"=w568, "format (%.3f)"="%.16f", "2D data"=w569, "append to file? (new file:F)"=TRUE ("append to file? (F)"), "transpose? (no:F)"=TRUE ("transpose? (F)")) -> ()  [unwired: 9 in, 2 out]
              n117 = call "Convert to Dynamic Data"("Array"=w571) -> ("Dynamic Data Type"=w579:dynamicdata)  [unwired: 3 in]
              n118 = call "Convert to Dynamic Data2"("Array"=w570) -> ("Dynamic Data Type"=w578:dynamicdata)  [unwired: 3 in]
              n119 = call "Build XY Graph"("Y Input"=w578, "X Input"=w579) -> ("XY Graph"=→"Spectrum":cluster{"Y":dbl[], "Y":dbl[]}[])  [unwired: 8 in, 1 out]
            }
            frame #8 {
              n120 = flat-sequence {
                frame #0 {
                  n121 = flat-sequence {
                    frame #0 {
                      n122 = call <vilib>:"Create Report.vi"("window state (normal)"=T3."no change", "report type"=Report_Type."Excel", "template (empty)"=path "D:/desktop/train/TEST1/Save/580中心波长.xlsx") -> ("report out"=w620:refnum<class "NI_report.lvclass">, "error out"=w619:errorcluster)  [unwired: 11 in]
                      n123 = call-poly <vilib>:"Excel Get Data.vi"("report in"=w620, "data type"=string[][] [], "error in (no error)"=w619) -> ("report out"=w615:refnum<class "NI_report.lvclass">, "data"=w622:string[][], "error out"=w614:errorcluster)  [unwired: 10 in]
                      n124 = call-dynamic "Dispose Report.vi"("report in"=w615, "error in (no error)"=w614) -> ()  [unwired: 13 in, 1 out]
                      n125 = Index Array(array=w622, index (col)=0 ("禁用的索引 (列)")) -> (element=w624:string[])  [unwired: 1 in]
                      n126 = Fract/Exp String To Number(string=w624) -> (number=w613:dbl[])  [unwired: 3 in, 1 out]
                      n127 = local write "波长范围"(w613) -> ()
                    }
                  }
                  n128 = local write "Target WL"("Target WL 2") -> ()
                }
                frame #1 {
                  n129 = local write "操作"(TRUE ("操作")) -> ()
                }
                frame #2 {
                  n130 = local write "Move To\nTarget Positions"(TRUE ("Move To\nTarget Positions")) -> ()
                  n131 = Wait (ms)(milliseconds to wait=u32 30000 ("等待时间（毫秒）")) -> ()  [unwired: 1 out]
                }
                frame #3 {
                  n132 = local write "Move To\nTarget Positions"(FALSE ("Move To\nTarget Positions")) -> ()
                }
                frame #4 {
                  n133 = local write "操作"(FALSE ("操作")) -> ()
                }
              }
            }
            frame #9 {
              (unwired) 0.0 ("元素")
              n134 = local read "Area Number to Display"() -> (w647:i32)
              n135 = local read "JYCCDLib.IJYCCDReqd"() -> (w643:refnum<k7>)
              n136 = call "MultiAccu - Acquire spectral.vi"("error in"=errorcluster {"status"=FALSE, "code"=0, "source"=""}, "Accumulations:"=u16 1, "ShutterOpen"=TRUE, "JYCCDLib.IJYCCDReqd"=w643) -> ("Acq Time(ms)"=w649:u32, "Array Out"=w648:i32[][][])  [unwired: 1 out]
              n137 = local write "Acq Time(ms)"(w649) -> ()
              n138 = local read "cut backlight"() -> (w638:bool)
              n139 = local read "backlight"() -> (w636:bool)
              n140 = And(x=w638, y=w636) -> (x .and. y?=w637:bool)
              n141 = call "Array reset dimension.vi"("Area Number"=w647, "Array In"=w648) -> ("Array Out"=w640:i32[][])
              n142 = case shown="真" w637 {
                tunnel: [w656 w658] -> w639
                tunnel: w640 -> [w656 w657]
                frame False {
                }
                frame True {
                  n143 = local read "Backlight"() -> (w659:i32[][])
                  n144 = Subtract(x=w657, y=w659) -> (x-y=w658:i32[][])
                }
              }
              n145 = local write "Data"(w640) -> ()
              n146 = local read "波长范围"() -> (w633:dbl[])
              n147 = Index Array(array=w639, index (row)=0 ("索引 (行)")) -> (element=w655:i32[])  [unwired: 1 in]
              n148 = Reverse 1D Array(array=w655) -> (reversed array=w635:i32[])
              n149 = call <vilib>:"Median Filter.vi"("left rank"=6, "X"=w635) -> ("Filtered X"=w632:dbl[])  [unwired: 8 in, 1 out]
              n150 = Build Array(w633, w632) -> (w631:dbl[][])
              n151 = call-poly <vilib>:"Write Delimited Spreadsheet.vi"("file path (dialog if empty)"=w630, "format (%.3f)"="%.16f", "2D data"=w631, "append to file? (new file:F)"=TRUE ("append to file? (F)"), "transpose? (no:F)"=TRUE ("transpose? (F)")) -> ()  [unwired: 9 in, 2 out]
              n152 = call "Convert to Dynamic Data5"("Array"=w633) -> ("Dynamic Data Type"=w642:dynamicdata)  [unwired: 3 in]
              n153 = call "Convert to Dynamic Data6"("Array"=w632) -> ("Dynamic Data Type"=w641:dynamicdata)  [unwired: 3 in]
              n154 = call "Build XY Graph4"("Y Input"=w641, "X Input"=w642) -> ("XY Graph"=w634:cluster{"Y":dbl[], "Y":dbl[]}[])  [unwired: 8 in, 1 out]
              n155 = local write "Spectrum"(w634) -> ()
            }
            frame #10 {
              n156 = flat-sequence {
                tunnel: w663 -> [w672]
                tunnel: w662 -> [w671]
                tunnel: [w667] -> w661
                tunnel: [w666] -> w660
                frame #0 {
                  n157 = local read "channel输出口"() -> (w665:i32)
                  n158 = case shown="1" w665 {
                    tunnel: [1 0] -> w664
                    frame 0, Default {
                    }
                    frame 1 {
                    }
                  }
                  n159 = local write "Output 2"(TRUE ("布尔")) -> ()
                  n160 = Pick Line(multi-line string=":OUTP1 ON\n:OUTP2 ON" ("write buffer"), line index=w664) -> (output string=w668:string)  [unwired: 1 in]
                  n161 = VISA Write(VISA resource name=w672, write buffer=w668, error in (no error)=w671) -> (VISA resource name out=w667:refnum<visa-resource-name>, error out=w666:errorcluster)  [unwired: 1 out]
                }
              }
            }
            frame #11 {
              w675 = " \u0001\u0000¡"  # Channel
              n162 = Concatenate Strings(w675, "\r") -> (w681:string)
              n163 = VISA Write(VISA resource name=w677, write buffer=w681, error in (no error)=w680) -> (VISA resource name out=w679:refnum<visa-resource-name>, error out=w678:errorcluster)  [unwired: 1 out]
              n164 = local write "照明光"(TRUE ("照明光")) -> ()
            }
            frame #12 {
              n165 = Wait (ms)(milliseconds to wait=900) -> ()  [unwired: 1 out]
            }
            frame #13 {
              n166 = Greater Or Equal?(x=w685, y=1) -> (x >= y?=w686:bool)
              n167 = case shown="真" w686 {
                tunnel: w688 -> [_ w693]
                tunnel: w687 -> [_ w694]
                frame False {
                }
                frame True {
                  n168 = local read "Δw1>C"() -> (w692:bool)
                  n169 = case shown="真" w692 {
                    tunnel: w694 -> [w703 _]
                    tunnel: w693 -> [w704 _]
                    frame False {
                      # "根据θ变化速度改变开光时间"
                      n170 = Subtract(x=w704, y=w703) -> (x-y=w706:dbl)
                      n171 = local read "开光时间/ms"() -> (w709:u32)
                      n172 = Absolute Value(x=w706) -> (abs(x)=w708:dbl)
                      n173 = Greater Or Equal?(x=w708, y="判断角度上限") -> (x >= y?=w707:bool)
                      n174 = case shown="假" w707 {
                        tunnel: w708 -> [w715 _]
                        tunnel: w709 -> [w712 w722]
                        tunnel: [w711 w720] -> w710
                        frame False {
                          n175 = Less Or Equal?(x=w715, y="判断角度下限") -> (x <= y?=w713:bool)
                          n176 = case shown="真" w713 {
                            tunnel: w712 -> [w716 w719]
                            tunnel: [w716 w718] -> w711
                            frame False {
                            }
                            frame True {
                              n177 = Multiply(x=w719, y="角度倍乘系数") -> (x*y=w718:dbl)
                            }
                          }
                        }
                        frame True {
                          n178 = Divide(x=w722, y=1.6) -> (x/y=w720:dbl)
                        }
                      }
                      n179 = local write "开光时间/ms"(w710) -> ()
                    }
                    frame True {
                    }
                  }
                  n180 = local read "Δw1>C"() -> (w690:bool)
                  n181 = local read "Δw2>C"() -> (w691:bool)
                  n182 = And(x=w690, y=w691) -> (x .and. y?=w689:bool)
                  n183 = case shown="真" w689 {
                    tunnel: w693 -> [_ w695]
                    frame False {
                    }
                    frame True {
                      # "4°后重置指示灯状态"
                      n184 = local read "θi"() -> (w699:dbl)
                      n185 = Subtract(x=w695, y=w699) -> (x-y=w700:dbl)
                      n186 = Absolute Value(x=w700) -> (abs(x)=w698:dbl)
                      n187 = Greater?(x=w698, y=15.0) -> (0:w696:bool)
                      n188 = case shown="真" w696 {
                        frame False {
                        }
                        frame True {
                          w701 = FALSE ("Δw1>C")
                          n189 = local write "Δw1>C"(w701) -> ()
                          n190 = local write "Δw2>C"(w701) -> ()
                          n191 = local write "θi"(0.0 ("θ")) -> ()
                        }
                      }
                    }
                  }
                }
              }
            }
            frame #14 {
              n192 = local write "正在测量"(FALSE) -> ()
            }
          }
        }
        n193 = VISA Close(VISA resource name=w414, error in (no error)=w413) -> (error out=→"output control error":errorcluster)
        n194 = VISA Close(VISA resource name=w417, error in (no error)=w416) -> (error out=→"照明光error out":errorcluster)
      }
    }
    n195 = flat-sequence {
      frame #0 {
        "Backlight" <- i32[][] [] ("Backlight")
      }
      frame #1 {
        w328 = FALSE
        # "删除背景光控件\n初始值设定"
        n196 = local write "cut backlight"(w328) -> ()
        "backlight" <- w328
      }
    }
    n197 = event shown="[1] \"Enable\": 值改变" {
      selector: _ -> [_ _]
      dyn-events: _ -> [_ _]
      timeout: u32 0 ("Time") -> [_ _]
      tunnel: "Enable" -> [_ w728]
      event Timeout {
        n198 = event-data() -> ()  [unwired: 1 in, 2 out]
      }
      event "Enable": Value Change {
        n199 = event-data() -> ()  [unwired: 1 in, 6 out]
        n200 = local read "VISA 信号发生器"() -> (w724:refnum<visa-resource-name>)
        n201 = VISA Open(VISA resource name=w724) -> (VISA resource name=w727:refnum<visa-resource-name>, error out=w730:errorcluster)  [unwired: 4 in]
        n202 = stacked-sequence {
          tunnel: w728 -> [w735 _]
          tunnel: w730 -> [w734 _]
          tunnel: w727 -> [w733 _]
          tunnel: [w732 _] -> w726
          tunnel: [w731 _] -> w725
          frame #0 {
            n203 = case shown="真" w735 {
              tunnel: w733 -> [w743 w751]
              tunnel: [w742 w750] -> w731
              tunnel: w734 -> [w741 w748]
              tunnel: [w740 w749] -> w732
              frame True {
                n204 = local write "Output"(TRUE ("布尔")) -> ()
                n205 = local read "channel输出口"() -> (w737:i32)
                n206 = Pick Line(multi-line string=":OUTP1 ON\n:OUTP2 ON" ("write buffer"), line index=w737) -> (output string=w736:string)  [unwired: 1 in]
                n207 = VISA Write(VISA resource name=w743, write buffer=w736, error in (no error)=w741) -> (VISA resource name out=w740:refnum<visa-resource-name>, error out=w742:errorcluster)  [unwired: 1 out]
              }
              frame False {
                n208 = local read "channel输出口"() -> (w745:i32)
                n209 = Pick Line(multi-line string=":OUTP1 OFF\n:OUTP2 OFF" ("write buffer"), line index=w745) -> (output string=w744:string)  [unwired: 1 in]
                n210 = VISA Write(VISA resource name=w751, write buffer=w744, error in (no error)=w748) -> (VISA resource name out=w749:refnum<visa-resource-name>, error out=w750:errorcluster)  [unwired: 1 out]
                n211 = local write "Output"(FALSE ("布尔")) -> ()
              }
            }
          }
          frame #1 {
            n212 = Wait (ms)(milliseconds to wait=u32 150) -> ()  [unwired: 1 out]
          }
        }
        n213 = VISA Close(VISA resource name=w726, error in (no error)=w725) -> (error out=→"output control error  5":errorcluster)
      }
    }
    n214 = event shown="[1] \"Enable 2\": 值改变" {
      selector: _ -> [_ _]
      dyn-events: _ -> [_ _]
      timeout: u32 0 ("Time") -> [_ _]
      tunnel: "Enable 2" -> [_ w330]
      event Timeout {
        n215 = event-data() -> ()  [unwired: 1 in, 2 out]
      }
      event "Enable 2": Value Change {
        n216 = event-data() -> ()  [unwired: 1 in, 6 out]
        n217 = Not(x=w330) -> (.not. x?=w329:bool)
        n218 = local read "VISA 信号发生器"() -> (w331:refnum<visa-resource-name>)
        n219 = VISA Open(VISA resource name=w331) -> (VISA resource name=w334:refnum<visa-resource-name>, error out=w335:errorcluster)  [unwired: 4 in]
        n220 = stacked-sequence {
          tunnel: w329 -> [w340 _]
          tunnel: w335 -> [w339 _]
          tunnel: w334 -> [w338 _]
          tunnel: [w337 _] -> w333
          tunnel: [w336 _] -> w332
          frame #0 {
            n221 = case shown="真" w340 {
              tunnel: w338 -> [w349 w360]
              tunnel: [w348 w359] -> w336
              tunnel: w339 -> [w347 w357]
              tunnel: [w346 w358] -> w337
              frame True {
                n222 = local read "channel输出口"() -> (w342:i32)
                n223 = local write "Output 2"(FALSE ("布尔")) -> ()
                n224 = case shown="1" w342 {
                  tunnel: [1 0] -> w341
                  frame 0, Default {
                  }
                  frame 1 {
                  }
                }
                n225 = Pick Line(multi-line string=":OUTP1 ON\n:OUTP2 ON" ("write buffer"), line index=w341) -> (output string=w343:string)  [unwired: 1 in]
                n226 = VISA Write(VISA resource name=w349, write buffer=w343, error in (no error)=w347) -> (VISA resource name out=w346:refnum<visa-resource-name>, error out=w348:errorcluster)  [unwired: 1 out]
              }
              frame False {
                n227 = local read "channel输出口"() -> (w353:i32)
                n228 = case shown="1" w353 {
                  tunnel: [1 0] -> w352
                  frame 0, Default {
                  }
                  frame 1 {
                  }
                }
                n229 = Pick Line(multi-line string=":OUTP1 OFF\n:OUTP2 OFF" ("write buffer"), line index=w352) -> (output string=w354:string)  [unwired: 1 in]
                n230 = VISA Write(VISA resource name=w360, write buffer=w354, error in (no error)=w357) -> (VISA resource name out=w358:refnum<visa-resource-name>, error out=w359:errorcluster)  [unwired: 1 out]
                n231 = local write "Output 2"(TRUE ("布尔")) -> ()
              }
            }
          }
          frame #1 {
            n232 = Wait (ms)(milliseconds to wait=u32 150) -> ()  [unwired: 1 out]
          }
        }
        n233 = VISA Close(VISA resource name=w333, error in (no error)=w332) -> ()  [unwired: 1 out]
      }
    }
    n234 = event shown="[1] \"低电平持续输出\": 值改变" {
      selector: _ -> [_ _]
      dyn-events: _ -> [_ _]
      timeout: u32 0 ("Time") -> [_ _]
      tunnel: "低电平持续输出" -> [_ w753]
      event Timeout {
        n235 = event-data() -> ()  [unwired: 1 in, 2 out]
      }
      event "低电平持续输出": Value Change {
        w757 = " :SOUR1\n :SOUR2"  # Channel
        n236 = event-data() -> ()  [unwired: 1 in, 6 out]
        n237 = local read "channel输出口"() -> (w758:i32)
        n238 = Pick Line(multi-line string=w757, line index=w758) -> (output string=w756:string)  [unwired: 1 in]
        n239 = local read "VISA 信号发生器"() -> (w761:refnum<visa-resource-name>)
        n240 = VISA Open(VISA resource name=w761) -> (VISA resource name=w760:refnum<visa-resource-name>, error out=w759:errorcluster)  [unwired: 4 in]
        n241 = stacked-sequence {
          seq-local: [w767 _ _ _ _ _ _ _ _ _ _ _ _] -> [_ _ w782 _ _ _ _ _ _ _ _ _ _]
          seq-local: [w766 _ _ _ _ _ _ _ _ _ _ _ _] -> [_ _ w781 _ _ _ _ _ _ _ _ _ _]
          seq-local: [_ _ w780 _ _ _ _ _ _ _ _ _ _] -> [_ _ _ _ w785 _ _ _ _ _ _ _ _]
          seq-local: [_ _ w779 _ _ _ _ _ _ _ _ _ _] -> [_ _ _ _ w786 _ _ _ _ _ _ _ _]
          seq-local: [_ _ _ _ w794 _ _ _ _ _ _ _ _] -> [_ _ _ _ _ _ w805 _ _ _ _ _ _]
          seq-local: [_ _ _ _ w793 _ _ _ _ _ _ _ _] -> [_ _ _ _ _ _ w804 _ _ _ _ _ _]
          seq-local: [_ _ _ _ _ _ w798 _ _ _ _ _ _] -> [_ _ _ _ _ _ _ _ w808 _ _ _ _]
          seq-local: [_ _ _ _ _ _ w797 _ _ _ _ _ _] -> [_ _ _ _ _ _ _ _ w807 _ _ _ _]
          seq-local: [_ _ _ _ _ _ _ _ w811 _ _ _ _] -> [_ _ _ _ _ _ _ _ _ _ w822 _ _]
          seq-local: [_ _ _ _ _ _ _ _ w810 _ _ _ _] -> [_ _ _ _ _ _ _ _ _ _ w821 _ _]
          seq-local: [_ _ _ _ _ _ _ _ _ _ w819 _ _] -> [_ _ _ _ _ _ _ _ _ _ _ _ w836]
          seq-local: [_ _ _ _ _ _ _ _ _ _ w818 _ _] -> [_ _ _ _ _ _ _ _ _ _ _ _ w835]
          tunnel: w760 -> [w772 _ _ _ _ _ _ _ _ _ _ _ _]
          tunnel: w759 -> [w765 _ _ _ _ _ _ _ _ _ _ _ _]
          tunnel: w756 -> [w764 _ w778 _ w791 _ w802 _ w812 _ w825 _ _]
          tunnel: [_ _ _ _ _ _ _ _ _ _ _ _ w834] -> w755
          tunnel: [_ _ _ _ _ _ _ _ _ _ _ _ w832] -> w754
          tunnel: w753 -> [_ _ _ _ _ _ _ _ _ _ _ _ w833]
          frame #0 {
            w769 = " PULSe"  # Function Command
            n242 = local read "输出信号波形"() -> (w763:u16)
            n243 = Concatenate Strings(w764, ":FUNC" ("string (\"\")")) -> (w770:string)
            n244 = Pick Line(string ("")=w770, multi-line string=w769, line index=w763) -> (output string=w768:string)
            n245 = VISA Write(VISA resource name=w772, write buffer=w768, error in (no error)=w765) -> (VISA resource name out=w767:refnum<visa-resource-name>, error out=w766:errorcluster)  [unwired: 1 out]
          }
          frame #1 {
            n246 = Wait (ms)(milliseconds to wait=u32 150) -> ()  [unwired: 1 out]
          }
          frame #2 {
            n247 = Number To Fractional String(use system decimal point (T)=TRUE ("使用系统小数点(T)"), number=1.0 ("数字")) -> (F-format string=w776:string)  [unwired: 2 in]
            n248 = Concatenate Strings ("连接字符串")(w778, ":VOLTage：HIGH ", w776) -> (w775:string)
            n249 = VISA Write(VISA resource name=w782, write buffer=w775, error in (no error)=w781) -> (VISA resource name out=w780:refnum<visa-resource-name>, error out=w779:errorcluster)  [unwired: 1 out]
          }
          frame #3 {
            n250 = Wait (ms)(milliseconds to wait=u32 150) -> ()  [unwired: 1 out]
          }
          frame #4 {
            # "1 电压偏置"
            n251 = Number To Fractional String(use system decimal point (T)=TRUE ("使用系统小数点(T)"), number=0.0 ("数字")) -> (F-format string=w789:string)  [unwired: 2 in]
            n252 = Concatenate Strings(w791, ":VOLTage:LOW ", w789) -> (w790:string)
            n253 = VISA Write(VISA resource name=w785, write buffer=w790, error in (no error)=w786) -> (VISA resource name out=w794:refnum<visa-resource-name>, error out=w793:errorcluster)  [unwired: 1 out]
          }
          frame #5 {
            n254 = Wait (ms)(milliseconds to wait=u32 150) -> ()  [unwired: 1 out]
          }
          frame #6 {
            n255 = local read "channel输出口"() -> (w800:i32)
            n256 = Pick Line(multi-line string=":OUTP1:IMPedance \n:OUTP2:IMPedance " ("write buffer"), line index=w800) -> (output string=w799:string)  [unwired: 1 in]
            n257 = Concatenate Strings ("连接字符串")(w802, w799, "INFINITY") -> (w803:string)
            n258 = VISA Write(VISA resource name=w805, write buffer=w803, error in (no error)=w804) -> (VISA resource name out=w798:refnum<visa-resource-name>, error out=w797:errorcluster)  [unwired: 1 out]
          }
          frame #7 {
            n259 = Wait (ms)(milliseconds to wait=u32 150) -> ()  [unwired: 1 out]
          }
          frame #8 {
            n260 = Number To Fractional String(use system decimal point (T)=TRUE ("使用系统小数点(T)"), number=0.0 ("数字")) -> (F-format string=w815:string)  [unwired: 2 in]
            n261 = Concatenate Strings(w812, ":PULSe:DELay ", w815) -> (w813:string)
            n262 = VISA Write(VISA resource name=w808, write buffer=w813, error in (no error)=w807) -> (VISA resource name out=w811:refnum<visa-resource-name>, error out=w810:errorcluster)  [unwired: 1 out]
          }
          frame #9 {
            n263 = Wait (ms)(milliseconds to wait=u32 150) -> ()  [unwired: 1 out]
          }
          frame #10 {
            w826 = ":LEADing\n:TRAiling "  # Channel
            w830 = ":PULSe:TRANsition"  # VOLTage:Offset
            n264 = local read "上升下降沿"() -> (w827:i32)
            n265 = Pick Line(multi-line string=w826, line index=w827) -> (output string=w823:string)  [unwired: 1 in]
            n266 = Number To Fractional String(use system decimal point (T)=TRUE ("使用系统小数点(T)"), number=0.0 ("数字")) -> (F-format string=w824:string)  [unwired: 2 in]
            n267 = Concatenate Strings(w825, w830, w823, w824) -> (w828:string)
            n268 = VISA Write(VISA resource name=w822, write buffer=w828, error in (no error)=w821) -> (VISA resource name out=w819:refnum<visa-resource-name>, error out=w818:errorcluster)  [unwired: 1 out]
          }
          frame #11 {
            n269 = Wait (ms)(milliseconds to wait=u32 150) -> ()  [unwired: 1 out]
          }
          frame #12 {
            n270 = case shown="假" w833 {
              tunnel: w836 -> [w844 w845]
              tunnel: [w843 w852] -> w832
              tunnel: w835 -> [w842 w850]
              tunnel: [w841 w851] -> w834
              frame True {
                n271 = local write "Output"(TRUE ("布尔")) -> ()
                n272 = local read "channel输出口"() -> (w838:i32)
                n273 = Pick Line(multi-line string=":OUTP1 ON\n:OUTP2 ON" ("write buffer"), line index=w838) -> (output string=w837:string)  [unwired: 1 in]
                n274 = VISA Write(VISA resource name=w844, write buffer=w837, error in (no error)=w842) -> (VISA resource name out=w841:refnum<visa-resource-name>, error out=w843:errorcluster)  [unwired: 1 out]
              }
              frame False {
                n275 = local read "channel输出口"() -> (w847:i32)
                n276 = Pick Line(multi-line string=":OUTP1 OFF\n:OUTP2 OFF" ("write buffer"), line index=w847) -> (output string=w846:string)  [unwired: 1 in]
                n277 = VISA Write(VISA resource name=w845, write buffer=w846, error in (no error)=w850) -> (VISA resource name out=w851:refnum<visa-resource-name>, error out=w852:errorcluster)  [unwired: 1 out]
                n278 = local write "Output"(FALSE ("布尔")) -> ()
              }
            }
          }
        }
        n279 = VISA Close(VISA resource name=w755, error in (no error)=w754) -> (error out=→"output control error  4":errorcluster)
      }
    }
    n280 = case shown="真" "设置参数" {
      frame False {
      }
      frame True {
        w859 = " :SOUR1\n :SOUR2"  # Channel
        n281 = local read "VISA 信号发生器"() -> (w861:refnum<visa-resource-name>)
        n282 = local read "channel输出口"() -> (w860:i32)
        n283 = case shown="1" w860 {
          tunnel: [1 0] -> w853
          frame 0, Default {
          }
          frame 1 {
          }
        }
        n284 = VISA Open(VISA resource name=w861) -> (VISA resource name=w864:refnum<visa-resource-name>, error out=w865:errorcluster)  [unwired: 4 in]
        n285 = Pick Line(multi-line string=w859, line index=w853) -> (output string=w854:string)  [unwired: 1 in]
        n286 = Pick Line(multi-line string=w859, line index=w860) -> (output string=w862:string)  [unwired: 1 in]
        n287 = stacked-sequence {
          seq-local: [w961 _ _ _ _ _ _ _ _ _ _ _ _ _ _] -> [_ _ w976 _ _ _ _ _ _ _ _ _ _ _ _]
          seq-local: [w960 _ _ _ _ _ _ _ _ _ _ _ _ _ _] -> [_ _ w975 _ _ _ _ _ _ _ w1014 _ _ _ _]
          seq-local: [_ _ w974 _ _ _ _ _ _ _ _ _ _ _ _] -> [_ _ _ _ w985 _ _ _ _ _ _ _ _ _ _]
          seq-local: [_ _ w973 _ _ _ _ _ _ _ _ _ _ _ _] -> [_ _ _ _ w984 _ _ _ _ _ _ _ _ _ _]
          seq-local: [_ _ _ _ w983 _ _ _ _ _ _ _ _ _ _] -> [_ _ _ _ _ _ w991 _ _ _ _ _ _ _ _]
          seq-local: [_ _ _ _ w980 _ _ _ _ _ _ _ _ _ _] -> [_ _ _ _ _ _ w990 _ _ _ _ _ _ _ _]
          seq-local: [_ _ _ _ _ _ w998 _ _ _ _ _ _ _ _] -> [_ _ _ _ _ _ _ _ w1009 _ _ _ _ _ _]
          seq-local: [_ _ _ _ _ _ w997 _ _ _ _ _ _ _ _] -> [_ _ _ _ _ _ _ _ w1008 _ _ _ _ _ _]
          seq-local: [_ _ _ _ _ _ _ _ w1002 _ _ _ _ _ _] -> [_ _ _ _ _ _ _ _ _ _ w1015 _ _ _ _]
          seq-local: [_ _ _ _ _ _ _ _ w1001 _ _ _ _ _ _] -> [_ _ _ _ _ _ _ _ _ _ _ _ _ _ _]
          seq-local: [_ _ _ _ _ _ _ _ _ _ w1011 _ _ _ _] -> [_ _ _ _ _ _ _ _ _ _ _ _ w1025 _ _]
          seq-local: [_ _ _ _ _ _ _ _ _ _ w1012 _ _ _ _] -> [_ _ _ _ _ _ _ _ _ _ _ _ w1024 _ _]
          seq-local: [_ _ _ _ _ _ _ _ _ _ _ _ w1023 _ _] -> [_ _ _ _ _ _ _ _ _ _ _ _ _ _ w1036]
          seq-local: [_ _ _ _ _ _ _ _ _ _ _ _ w1022 _ _] -> [_ _ _ _ _ _ _ _ _ _ _ _ _ _ w1035]
          tunnel: w864 -> [w966 _ _ _ _ _ _ _ _ _ _ _ _ _ _]
          tunnel: w865 -> [w959 _ _ _ _ _ _ _ _ _ _ _ _ _ _]
          tunnel: w862 -> [w958 _ w972 _ w979 _ w995 _ w1006 _ w1016 _ w1026 _ w1039]
          tunnel: [_ _ _ _ _ _ _ _ _ _ _ _ _ _ w1034] -> w858
          tunnel: [_ _ _ _ _ _ _ _ _ _ _ _ _ _ w1033] -> w857
          frame #0 {
            w963 = " PULSe"  # Function Command
            n288 = local read "输出信号波形"() -> (w957:u16)
            n289 = Concatenate Strings(w958, ":FUNC" ("string (\"\")")) -> (w964:string)
            n290 = Pick Line(string ("")=w964, multi-line string=w963, line index=w957) -> (output string=w962:string)
            n291 = VISA Write(VISA resource name=w966, write buffer=w962, error in (no error)=w959) -> (VISA resource name out=w961:refnum<visa-resource-name>, error out=w960:errorcluster)  [unwired: 1 out]
          }
          frame #1 {
            n292 = Wait (ms)(milliseconds to wait=u32 150) -> ()  [unwired: 1 out]
          }
          frame #2 {
            n293 = Number To Fractional String(use system decimal point (T)=TRUE ("使用系统小数点(T)"), number="低电平/V") -> (F-format string=w970:string)  [unwired: 2 in]
            n294 = Concatenate Strings ("连接字符串")(w972, ":VOLTage:LOW ", w970) -> (w969:string)
            n295 = VISA Write(VISA resource name=w976, write buffer=w969, error in (no error)=w975) -> (VISA resource name out=w974:refnum<visa-resource-name>, error out=w973:errorcluster)  [unwired: 1 out]
          }
          frame #3 {
            n296 = Wait (ms)(milliseconds to wait=u32 150) -> ()  [unwired: 1 out]
          }
          frame #4 {
            # "1 频率"
            n297 = Concatenate Strings(w979, ":FREQ ") -> (w986:string)
            n298 = Format Into String ("格式化写入字符串")(initial string=w986, "频率/Hz") -> (resulting string=w987:string)  [unwired: 2 in, 1 out]
            n299 = VISA Write(VISA resource name=w985, write buffer=w987, error in (no error)=w984) -> (VISA resource name out=w983:refnum<visa-resource-name>, error out=w980:errorcluster)  [unwired: 1 out]
          }
          frame #5 {
            n300 = Wait (ms)(milliseconds to wait=u32 150) -> ()  [unwired: 1 out]
          }
          frame #6 {
            n301 = Number To Fractional String(use system decimal point (T)=TRUE ("使用系统小数点(T)"), number="高电平/V") -> (F-format string=w992:string)  [unwired: 2 in]
            n302 = Concatenate Strings(w995, ":VOLTage:HIGH ", w992) -> (w994:string)
            n303 = VISA Write(VISA resource name=w991, write buffer=w994, error in (no error)=w990) -> (VISA resource name out=w998:refnum<visa-resource-name>, error out=w997:errorcluster)  [unwired: 1 out]
          }
          frame #7 {
            n304 = Wait (ms)(milliseconds to wait=u32 150) -> ()  [unwired: 1 out]
          }
          frame #8 {
            n305 = local read "channel输出口"() -> (w1004:i32)
            n306 = Pick Line(multi-line string=":OUTP1:IMPedance \n:OUTP2:IMPedance " ("write buffer"), line index=w1004) -> (output string=w1003:string)  [unwired: 1 in]
            n307 = Concatenate Strings ("连接字符串")(w1006, w1003, "INFINITY") -> (w1007:string)
            n308 = VISA Write(VISA resource name=w1009, write buffer=w1007, error in (no error)=w1008) -> (VISA resource name out=w1002:refnum<visa-resource-name>, error out=w1001:errorcluster)  [unwired: 1 out]
          }
          frame #9 {
            n309 = Wait (ms)(milliseconds to wait=u32 150) -> ()  [unwired: 1 out]
          }
          frame #10 {
            n310 = Number To Fractional String(use system decimal point (T)=TRUE ("使用系统小数点(T)"), number="占空比/%") -> (F-format string=w1018:string)  [unwired: 2 in]
            n311 = Concatenate Strings(w1016, ":PULSe:DCYCle ", w1018) -> (w1013:string)
            n312 = VISA Write(VISA resource name=w1015, write buffer=w1013, error in (no error)=w1014) -> (VISA resource name out=w1011:refnum<visa-resource-name>, error out=w1012:errorcluster)  [unwired: 1 out]
          }
          frame #11 {
            n313 = Wait (ms)(milliseconds to wait=u32 150) -> ()  [unwired: 1 out]
          }
          frame #12 {
            n314 = Number To Fractional String(use system decimal point (T)=TRUE ("使用系统小数点(T)"), number="延时/s") -> (F-format string=w1029:string)  [unwired: 2 in]
            n315 = Concatenate Strings(w1026, ":PULSe:DELay ", w1029) -> (w1027:string)
            n316 = VISA Write(VISA resource name=w1025, write buffer=w1027, error in (no error)=w1024) -> (VISA resource name out=w1023:refnum<visa-resource-name>, error out=w1022:errorcluster)  [unwired: 1 out]
          }
          frame #13 {
            n317 = Wait (ms)(milliseconds to wait=u32 150) -> ()  [unwired: 1 out]
          }
          frame #14 {
            w1040 = ":LEADing\n:TRAiling "  # Channel
            w1045 = ":PULSe:TRANsition"  # VOLTage:Offset
            n318 = local read "上升下降沿"() -> (w1041:i32)
            n319 = Pick Line(multi-line string=w1040, line index=w1041) -> (output string=w1037:string)  [unwired: 1 in]
            n320 = Number To Fractional String(use system decimal point (T)=TRUE ("使用系统小数点(T)"), number="上升下降沿/s") -> (F-format string=w1038:string)  [unwired: 2 in]
            n321 = Concatenate Strings(w1039, w1045, w1037, w1038) -> (w1042:string)
            n322 = VISA Write(VISA resource name=w1036, write buffer=w1042, error in (no error)=w1035) -> (VISA resource name out=w1034:refnum<visa-resource-name>, error out=w1033:errorcluster)  [unwired: 1 out]
          }
        }
        n323 = stacked-sequence {
          seq-local: [w872 _ _ _ _ _ _ _ _ _ _ _ _ _ _] -> [_ _ w887 _ _ _ _ _ _ _ _ _ _ _ _]
          seq-local: [w871 _ _ _ _ _ _ _ _ _ _ _ _ _ _] -> [_ _ w886 _ _ _ _ _ _ _ w925 _ _ _ _]
          seq-local: [_ _ w885 _ _ _ _ _ _ _ _ _ _ _ _] -> [_ _ _ _ w896 _ _ _ _ _ _ _ _ _ _]
          seq-local: [_ _ w884 _ _ _ _ _ _ _ _ _ _ _ _] -> [_ _ _ _ w895 _ _ _ _ _ _ _ _ _ _]
          seq-local: [_ _ _ _ w894 _ _ _ _ _ _ _ _ _ _] -> [_ _ _ _ _ _ w902 _ _ _ _ _ _ _ _]
          seq-local: [_ _ _ _ w891 _ _ _ _ _ _ _ _ _ _] -> [_ _ _ _ _ _ w901 _ _ _ _ _ _ _ _]
          seq-local: [_ _ _ _ _ _ w909 _ _ _ _ _ _ _ _] -> [_ _ _ _ _ _ _ _ w920 _ _ _ _ _ _]
          seq-local: [_ _ _ _ _ _ w908 _ _ _ _ _ _ _ _] -> [_ _ _ _ _ _ _ _ w919 _ _ _ _ _ _]
          seq-local: [_ _ _ _ _ _ _ _ w914 _ _ _ _ _ _] -> [_ _ _ _ _ _ _ _ _ _ w926 _ _ _ _]
          seq-local: [_ _ _ _ _ _ _ _ w913 _ _ _ _ _ _] -> [_ _ _ _ _ _ _ _ _ _ _ _ _ _ _]
          seq-local: [_ _ _ _ _ _ _ _ _ _ w922 _ _ _ _] -> [_ _ _ _ _ _ _ _ _ _ _ _ w936 _ _]
          seq-local: [_ _ _ _ _ _ _ _ _ _ w923 _ _ _ _] -> [_ _ _ _ _ _ _ _ _ _ _ _ w935 _ _]
          seq-local: [_ _ _ _ _ _ _ _ _ _ _ _ w934 _ _] -> [_ _ _ _ _ _ _ _ _ _ _ _ _ _ w949]
          seq-local: [_ _ _ _ _ _ _ _ _ _ _ _ w933 _ _] -> [_ _ _ _ _ _ _ _ _ _ _ _ _ _ w948]
          tunnel: w858 -> [w877 _ _ _ _ _ _ _ _ _ _ _ _ _ _]
          tunnel: w857 -> [w870 _ _ _ _ _ _ _ _ _ _ _ _ _ _]
          tunnel: w854 -> [w869 _ w883 _ w890 _ w906 _ w917 _ w927 _ w937 _ w944]
          tunnel: [_ _ _ _ _ _ _ _ _ _ _ _ _ _ w947] -> w856
          tunnel: [_ _ _ _ _ _ _ _ _ _ _ _ _ _ w946] -> w855
          tunnel: w853 -> [_ _ _ _ _ _ _ _ w911 _ _ _ _ _ _]
          frame #0 {
            w874 = " PULSe"  # Function Command
            n324 = Concatenate Strings(w869, ":FUNC" ("string (\"\")")) -> (w875:string)
            n325 = Pick Line(string ("")=w875, multi-line string=w874, line index="输出信号波形 2") -> (output string=w873:string)
            n326 = VISA Write(VISA resource name=w877, write buffer=w873, error in (no error)=w870) -> (VISA resource name out=w872:refnum<visa-resource-name>, error out=w871:errorcluster)  [unwired: 1 out]
          }
          frame #1 {
            n327 = Wait (ms)(milliseconds to wait=u32 150) -> ()  [unwired: 1 out]
          }
          frame #2 {
            n328 = Number To Fractional String(use system decimal point (T)=TRUE ("使用系统小数点(T)"), number="低电平/V 2") -> (F-format string=w881:string)  [unwired: 2 in]
            n329 = Concatenate Strings ("连接字符串")(w883, ":VOLTage:LOW ", w881) -> (w880:string)
            n330 = VISA Write(VISA resource name=w887, write buffer=w880, error in (no error)=w886) -> (VISA resource name out=w885:refnum<visa-resource-name>, error out=w884:errorcluster)  [unwired: 1 out]
          }
          frame #3 {
            n331 = Wait (ms)(milliseconds to wait=u32 150) -> ()  [unwired: 1 out]
          }
          frame #4 {
            # "1 频率"
            n332 = Concatenate Strings(w890, ":FREQ ") -> (w897:string)
            n333 = Format Into String ("格式化写入字符串")(initial string=w897, "频率/Hz 2") -> (resulting string=w898:string)  [unwired: 2 in, 1 out]
            n334 = VISA Write(VISA resource name=w896, write buffer=w898, error in (no error)=w895) -> (VISA resource name out=w894:refnum<visa-resource-name>, error out=w891:errorcluster)  [unwired: 1 out]
          }
          frame #5 {
            n335 = Wait (ms)(milliseconds to wait=u32 150) -> ()  [unwired: 1 out]
          }
          frame #6 {
            n336 = Number To Fractional String(use system decimal point (T)=TRUE ("使用系统小数点(T)"), number="高电平/V 2") -> (F-format string=w903:string)  [unwired: 2 in]
            n337 = Concatenate Strings(w906, ":VOLTage:HIGH ", w903) -> (w905:string)
            n338 = VISA Write(VISA resource name=w902, write buffer=w905, error in (no error)=w901) -> (VISA resource name out=w909:refnum<visa-resource-name>, error out=w908:errorcluster)  [unwired: 1 out]
          }
          frame #7 {
            n339 = Wait (ms)(milliseconds to wait=u32 150) -> ()  [unwired: 1 out]
          }
          frame #8 {
            n340 = Pick Line(multi-line string=":OUTP1:IMPedance \n:OUTP2:IMPedance " ("write buffer"), line index=w911) -> (output string=w915:string)  [unwired: 1 in]
            n341 = Concatenate Strings ("连接字符串")(w917, w915, "INFINITY") -> (w918:string)
            n342 = VISA Write(VISA resource name=w920, write buffer=w918, error in (no error)=w919) -> (VISA resource name out=w914:refnum<visa-resource-name>, error out=w913:errorcluster)  [unwired: 1 out]
          }
          frame #9 {
            n343 = Wait (ms)(milliseconds to wait=u32 150) -> ()  [unwired: 1 out]
          }
          frame #10 {
            n344 = Number To Fractional String(use system decimal point (T)=TRUE ("使用系统小数点(T)"), number="占空比/% 2") -> (F-format string=w929:string)  [unwired: 2 in]
            n345 = Concatenate Strings(w927, ":PULSe:DCYCle ", w929) -> (w924:string)
            n346 = VISA Write(VISA resource name=w926, write buffer=w924, error in (no error)=w925) -> (VISA resource name out=w922:refnum<visa-resource-name>, error out=w923:errorcluster)  [unwired: 1 out]
          }
          frame #11 {
            n347 = Wait (ms)(milliseconds to wait=u32 150) -> ()  [unwired: 1 out]
          }
          frame #12 {
            n348 = Number To Fractional String(use system decimal point (T)=TRUE ("使用系统小数点(T)"), number="延时/s 2") -> (F-format string=w940:string)  [unwired: 2 in]
            n349 = Concatenate Strings(w937, ":PULSe:DELay ", w940) -> (w938:string)
            n350 = VISA Write(VISA resource name=w936, write buffer=w938, error in (no error)=w935) -> (VISA resource name out=w934:refnum<visa-resource-name>, error out=w933:errorcluster)  [unwired: 1 out]
          }
          frame #13 {
            n351 = Wait (ms)(milliseconds to wait=u32 150) -> ()  [unwired: 1 out]
          }
          frame #14 {
            w952 = ":LEADing\n:TRAiling "  # Channel
            w956 = ":PULSe:TRANsition"  # VOLTage:Offset
            n352 = Pick Line(multi-line string=w952, line index="上升下降沿 2") -> (output string=w950:string)  [unwired: 1 in]
            n353 = Number To Fractional String(use system decimal point (T)=TRUE ("使用系统小数点(T)"), number="上升下降沿/s 2") -> (F-format string=w951:string)  [unwired: 2 in]
            n354 = Concatenate Strings(w944, w956, w950, w951) -> (w953:string)
            n355 = VISA Write(VISA resource name=w949, write buffer=w953, error in (no error)=w948) -> (VISA resource name out=w947:refnum<visa-resource-name>, error out=w946:errorcluster)  [unwired: 1 out]
          }
        }
        n356 = VISA Close(VISA resource name=w856, error in (no error)=w855) -> (error out=→"configure error out":errorcluster)
      }
    }
    n357 = case shown="真" "操作" {
      frame False {
      }
      frame True {
        n358 = stacked-sequence {
          seq-local: [_ _ _ w47 _ _ _ _] -> [_ _ _ _ w65 w85 w88 w237]
          seq-local: [_ _ _ w46 _ _ _ _] -> [_ _ _ _ w66 w86 w87 w238]
          frame #0 {
            # "initialize all variables"
            n359 = property on="initialize" class="Bool"("Désactivé"=u8 0) -> ()  [unwired: 2 in, 2 out]
            n360 = property on="Acquire" class="Bool"("Visible"=FALSE) -> ()  [unwired: 2 in, 2 out]
            n361 = property on="Setup" class="Bool"("Visible"=FALSE) -> ()  [unwired: 2 in, 2 out]
            n362 = local write "indicator"("" ("indicator")) -> ()
            n363 = local write "initialized ?"(FALSE ("initialized ?")) -> ()
            n364 = local write "Continuous"(FALSE ("Continuous")) -> ()
            n365 = local write "Close"(FALSE ("Close")) -> ()
            n366 = property on="Device Name" class="Ring (严格)"("Désactivé"=u8 0) -> ()  [unwired: 2 in, 2 out]
            n367 = property on="Continuous" class="Bool (严格)"("Visible"=FALSE) -> ()  [unwired: 2 in, 2 out]
            n368 = local write "Commande tab"(T1."Settings" ("Commande tab")) -> ()
          }
          frame #1 {
            # "Read Uniq ID"
            n369 = stacked-sequence {
              frame #0 {
                n370 = call "read detector uniq-id.vi"() -> ("nbr of components"=w39:i32, "UniqueID"=w38:string[], "Name"=w37:string[])  [unwired: 4 out]
                n371 = for {
                  N: w39 -> [_]
                  tunnel: w38 -> [w41]
                  tunnel: w37 -> [w40]
                  n372 = property on="Device Name" class="Ring (严格)"("Chaînes []"=w40) -> ()  [unwired: 2 in, 2 out]
                  n373 = property on="Uniques ID" class="Ring (严格)"("Chaînes []"=w41) -> ()  [unwired: 2 in, 2 out]
                }
              }
            }
          }
          frame #2 {
            n374 = while {
              stop <- "initialize" stop-if-true
              n375 = local read "Device Name"() -> (w44:u16)
              n376 = local write "Uniques ID"(w44) -> ()
              n377 = local read "Close"() -> (w42:bool)
              n378 = Stop(stop? (T)=w42) -> ()
              n379 = Wait Until Next ms Multiple(millisecond multiple=u32 100 ("n millisecondes")) -> ()  [unwired: 1 out]
            }
          }
          frame #3 {
            n380 = stacked-sequence {
              tunnel: [_ w54 _ _] -> w47
              tunnel: [_ w53 _ _] -> w46
              frame #0 {
                n381 = local write "indicator"("Initializing ..." ("indicator")) -> ()
              }
              frame #1 {
                n382 = local read "Uniques ID"() -> (w51:u16)
                n383 = property on="Uniques ID" class="Ring (严格)"() -> ("Chaînes []"=w52:string[])  [unwired: 2 in, 2 out]
                n384 = Index Array(array=w52, index=w51) -> (element=w50:string)
                n385 = call "Initialize CCD.vi"("Unique id:"=w50) -> ("activeYPixels"=→"Y Pixels:":i32, "JYCCDLib.IJYCCDReqd"=w53:refnum<k7>, "activeXPixels"=→"X Pixels:":i32, "sortie d'erreur"=w54:errorcluster, "FirmwareVersion"=→"Firmware\nVersion":string)  [unwired: 3 out]
              }
              frame #2 {
                n386 = property on="initialize" class="Bool"("Désactivé"=u8 2) -> ()  [unwired: 2 in, 2 out]
                n387 = property on="Device Name" class="Ring (严格)"("Désactivé"=u8 2) -> ()  [unwired: 2 in, 2 out]
                n388 = local write "Continuous"(FALSE ("Continuous")) -> ()
                n389 = property on="Setup" class="Bool"("Visible"=TRUE) -> ()  [unwired: 2 in, 2 out]
              }
              frame #3 {
                n390 = local write "initialized ?"(TRUE ("initialized ?")) -> ()
                n391 = local write "indicator"("Initialized !" ("indicator")) -> ()
              }
            }
          }
          frame #4 {
            # "Actually not working"
            # "Read ADC and GAIN"
            n392 = case shown="真" "Constante de condition\n(Voir l'aide contextuelle)" {
              tunnel: w66 -> [_ w76]
              tunnel: w65 -> [_ w75]
              frame False {
              }
              frame True {
                # "Read Input supported trigger"
                n393 = call "Trigger - Get Supported Input.vi"("JYCCDLib.IJYCCDReqd"=w76, "Error Input"=w75) -> ("trigAddress"=w70:i32, "eventPtr"=w71:i32, "trigEventString"=w74:string, "trigSigType"=w73:i32, "trigSigTypeString"=w72:string)  [unwired: 4 out]
                n394 = local write "trigSigTypeString"(w72) -> ()
                n395 = local write "trigAddress"(w70) -> ()
                n396 = local write "Trigger Type :"(w71) -> ()
                n397 = local write "trigEventString"(w74) -> ()
                n398 = local write "Signal type :"(w73) -> ()
              }
            }
            n399 = call "Init ADC & Gain.vi"("JYCCDLib.IJYCCDReqd"=w66, "input error"=w65) -> ("ADC Number"=w64:i32[], "ADC description"=w69:string[], "Gain Number"=w67:i32[], "Gain description"=w68:string[])
            n400 = local write "Gain Number"(w67) -> ()
            n401 = local write "ADC Number"(w64) -> ()
            n402 = stacked-sequence {
              tunnel: w69 -> [w77 _]
              tunnel: w68 -> [_ w78]
              frame #0 {
                n403 = property on="ADC" class="Ring (严格)"("Chaînes []"=w77) -> ()  [unwired: 2 in, 2 out]
              }
              frame #1 {
                n404 = property on="GAIN" class="Ring (严格)"("Chaînes []"=w78) -> ()  [unwired: 2 in, 2 out]
              }
            }
          }
          frame #5 {
            # "IS multi Accumulation Supported ?"
            n405 = call "MultiAccu - Is Supported.vi"("Error In"=w85, "JYCCDLib.IJYCCDReqd"=w86) -> ("IsOperatingModeSupported"=w79:bool)  [unwired: 3 out]
            n406 = Select(t=0, s=w79, f=2) -> (s? t:f=w82:i32)
            n407 = Select(t=FALSE, s=w79, f=w79) -> (s? t:f=w81:bool)
            n408 = local write "Multi Accumulation mode:"(w81) -> ()
            n409 = property on="Multi Accumulation mode:" class="Bool (严格)"("Désactivé"=w82) -> ()  [unwired: 2 in, 2 out]
            n410 = property on="Multi Accumulation mode:" class="Bool (严格)"("Désactivé"=w82) -> ()  [unwired: 2 in, 2 out]
          }
          frame #6 {
            n411 = while {
              tunnel: w87 -> [w95]
              tunnel: w88 -> [w94]
              stop <- "Close" stop-if-true
              n412 = local read "Continuous"() -> (w96:bool)
              n413 = case shown="假" "Reformat" {
                frame False {
                }
                frame True {
                  n414 = local read "Y Pixels:"() -> (w215:i32)
                  n415 = local read "X Pixels:"() -> (w217:i32)
                  n416 = call "Spectral Reformat CCD area.vi"("Y Pixels:"=w215, "X Pixels:"=w217, "numAreas"="Number of Areas :") -> ("areas :"=→"areas :":i32[][])  [unwired: 3 out]
                }
              }
              n417 = local read "Accumulations:"() -> (w91:u16)
              n418 = Or(x="Acquire", y=w96) -> (x .or. y?=w93:bool)
              n419 = case shown="真" w93 {
                tunnel: w95 -> [_ w108]
                tunnel: w94 -> [_ w107]
                tunnel: "Enable InputTriggers :" -> [_ w106]
                tunnel: "Multi Accumulation mode:" -> [_ w105]
                tunnel: w91 -> [_ w104]
                tunnel: "MultiAcqShutterMode" -> [_ w103]
                frame False {
                }
                frame True {
                  n420 = stacked-sequence {
                    seq-local: [_ _ w121 _ _] -> [_ _ _ w176 _]
                    tunnel: w108 -> [_ w110 w125 w175 _]
                    tunnel: w107 -> [_ w111 w124 w174 _]
                    tunnel: w106 -> [_ w112 _ _ _]
                    tunnel: w105 -> [_ _ w123 _ _]
                    tunnel: w104 -> [_ _ w122 _ _]
                    tunnel: w103 -> [_ _ w120 _ _]
                    frame #0 {
                      n421 = local write "CCD Busy"(TRUE ("CCD Busy")) -> ()
                    }
                    frame #1 {
                      n422 = case shown="真" w112 {
                        tunnel: w111 -> [w113 w119]
                        tunnel: w110 -> [w114 w118]
                        frame False {
                          n423 = call "Trigger - Disable.vi"("Error In"=w113, "JYCCDLib.IJYCCDReqd"=w114) -> ()  [unwired: 6 out]
                        }
                        frame True {
                          n424 = local read "Trigger Type :"() -> (w115:u16)
                          n425 = local read "Signal type :"() -> (w116:enum16{"TTL Rising Edge", "TTL Falling Edge"})
                          n426 = local read "trigAddress"() -> (w117:i32)
                          n427 = call "Trigger - Enable.vi"("Error In"=w119, "sigType"=w116, "event"=w115, "trigAddress"=w117, "JYCCDLib.IJYCCDReqd"=w118) -> ()  [unwired: 3 out]
                        }
                      }
                    }
                    frame #2 {
                      n428 = case shown="真" w123 {
                        selector: w123 -> [_ w154]
                        tunnel: w125 -> [w151 w157]
                        tunnel: w124 -> [w150 w156]
                        tunnel: w122 -> [_ w155]
                        tunnel: [u16 1 ("Accumulations:") w155] -> w121
                        tunnel: w120 -> [_ w153]
                        frame False {
                          n429 = call "MultiAccu - Disable.vi"("Error In"=w150, "JYCCDLib.IJYCCDReqd"=w151) -> ()  [unwired: 4 out]
                        }
                        frame True {
                          n430 = call "MultiAccu - Configure.vi"("JYCCDLib.IJYCCDReqd"=w157, "Cleans Before"="Number of Cleans", "Accumulations:"=w155, "MultiAcqHardwareMode"=w154, "MultiAcqShutterMode"=w153, "Error In"=w156) -> ()  [unwired: 1 in, 9 out]
                        }
                      }
                      n431 = flat-sequence {
                        frame #0 {
                          n432 = Current VI's Path() -> (path=w131:path)
                          n433 = Get Date/Time In Seconds() -> (seconds since 1Jan1904=w133:timestamp)
                          n434 = Strip Path(path=w131) -> (stripped path=w132:path)  [unwired: 1 out]
                          n435 = Path To String(path=w132) -> (string=w134:string)
                          n436 = Format Date/Time String(time format string (%c)="%m.%d" ("时间格式字符串(%c)"), seconds (now)=w133) -> (date/time string=w140:string)  [unwired: 1 in]
                          n437 = Concatenate Strings(w134, "\\Save\\" ("字符串"), w140) -> (w135:string)
                          n438 = String To Path(string=w135) -> (path=w136:path)
                          n439 = call <vilib>:"Check if File or Folder Exists.vi"("path"=w136) -> ("file or folder exists?"=w137:bool, "dup path"=w139:path)  [unwired: 8 in, 1 out]
                          n440 = case shown="真" w137 {
                            tunnel: [w147 w148] -> w138
                            tunnel: w139 -> [w146 w148]
                            tunnel: w140 -> [w145 _]
                            frame False {
                              n441 = Create Folder(prompt (Create Folder)=w145, path (use dialog)=w146) -> (created path=w147:path)  [unwired: 1 in, 2 out]
                            }
                            frame True {
                            }
                          }
                          n442 = Format Date/Time String(time format string (%c)="%y%m%d%H%M%S " ("时间格式字符串(%c)"), seconds (now)=w133) -> (date/time string=w143:string)  [unwired: 1 in]
                          n443 = Path To String(path=w138) -> (string=w141:string)
                          n444 = Concatenate Strings(w141, "\\" ("字符串")) -> (w142:string)
                          n445 = Concatenate Strings(w142, w143) -> (w130:string)
                          n446 = String To Path(string=w130) -> (path=→"最终存储路径 2":path)
                        }
                      }
                    }
                    frame #3 {
                      n447 = local read "cut backlight"() -> (w163:bool)
                      n448 = local read "backlight"() -> (w162:bool)
                      n449 = call "MultiAccu - Acquire spectral.vi"("error in"=w174, "Accumulations:"=w176, "ShutterOpen"="ShutterOpen", "JYCCDLib.IJYCCDReqd"=w175) -> ("Acq Time(ms)"=→"Acq Time(ms)":u32, "Array Out"=w173:i32[][][])  [unwired: 1 out]
                      n450 = And(x=w163, y=w162) -> (x .and. y?=w164:bool)
                      n451 = call "Array reset dimension.vi"("Area Number"="Area Number to Display", "Array In"=w173) -> ("Array Out"=w165:i32[][])
                      n452 = case shown="真" w164 {
                        tunnel: [w179 w180] -> w166
                        tunnel: w165 -> [w179 w181]
                        frame False {
                        }
                        frame True {
                          n453 = local read "Backlight"() -> (w182:i32[][])
                          n454 = Subtract(x=w181, y=w182) -> (x-y=w180:i32[][])
                        }
                      }
                      n455 = local read "波长范围"() -> (w159:dbl[])
                      n456 = local write "Data"(w165) -> ()
                      n457 = Index Array(array=w166, index (row)=0 ("禁用的索引 (列)")) -> (element=w167:i32[])  [unwired: 1 in]
                      n458 = Reverse 1D Array(array=w167) -> (reversed array=w160:i32[])
                      n459 = call <vilib>:"Median Filter.vi"("left rank"=6, "X"=w160) -> ("Filtered X"=w158:dbl[])  [unwired: 8 in, 1 out]
                      n460 = call "转换至动态数据2"("Array"=w159) -> ("Dynamic Data Type"=w169:dynamicdata)  [unwired: 3 in]
                      n461 = call "转换至动态数据"("Array"=w158) -> ("Dynamic Data Type"=w170:dynamicdata)  [unwired: 3 in]
                      n462 = call "Build XY Graph2"("Y Input"=w170, "X Input"=w169) -> ("XY Graph"=w168:cluster{"Y":dbl[], "Y":dbl[]}[])  [unwired: 8 in, 1 out]
                      n463 = local write "Spectrum"(w168) -> ()
                    }
                    frame #4 {
                      n464 = case shown="真" "是否保存" {
                        frame False {
                        }
                        frame True {
                          n465 = Get Date/Time In Seconds() -> (seconds since 1Jan1904=w199:timestamp)
                          n466 = Get Date/Time String(date format (0)=enum16{"short", "long", "abbreviated"}."abbreviated" ("日期格式(0)"), seconds (now)=w199, want seconds? (F)=TRUE ("需要秒？(F)")) -> (date string=w197:string, time string=w198:string)
                          n467 = Search and Replace String(replace all?=TRUE ("替换全部？(F)"), input string=w198, search string=":" ("搜索字符串"), replace string="-" ("替换字符串(\"\")")) -> (result string=w196:string)  [unwired: 4 in, 3 out]
                          n468 = local read "最终存储路径 2"() -> (w200:path)
                          n469 = Path To String(path=w200) -> (string=w203:string)
                          n470 = Concatenate Strings(w203, w197, w196, "光谱" ("字符串"), ".xls" ("字符串")) -> (w202:string)
                          n471 = String To Path(string=w202) -> (path=w201:path)
                          n472 = call-poly <vilib>:"Write Delimited Spreadsheet.vi"("file path (dialog if empty)"=w201, "format (%.3f)"="%.16f", "append to file? (new file:F)"=TRUE ("append to file? (F)"), "transpose? (no:F)"=TRUE ("transpose? (F)")) -> ()  [unwired: 10 in, 2 out]
                        }
                      }
                      n473 = case shown="真" "Save Backlight" {
                        frame False {
                        }
                        frame True {
                          w204 = TRUE ("删除背景光")
                          n474 = local read "Data"() -> (w206:i32[][])
                          n475 = local write "Backlight"(w206) -> ()
                          n476 = local write "cut backlight"(w204) -> ()
                          n477 = local write "backlight"(w204) -> ()
                          n478 = local write "Save Backlight"(FALSE ("Save Backlight")) -> ()
                        }
                      }
                      n479 = local write "CCD Busy"(FALSE ("CCD Busy")) -> ()
                    }
                  }
                }
              }
              n480 = case shown="假" "Setup" {
                tunnel: w94 -> [_ w220]
                tunnel: w95 -> [_ w219]
                frame False {
                }
                frame True {
                  n481 = stacked-sequence {
                    tunnel: w220 -> [_ w234 _]
                    tunnel: w219 -> [_ w222 _]
                    frame #0 {
                      n482 = local write "indicator"("Setting up the detector" ("indicator")) -> ()
                    }
                    frame #1 {
                      w232 = 1 items=["JYMCD_ACQ_FORMAT_IMAGE", "JYMCD_ACQ_FORMAT_SCAN"] ("Acquisition type")
                      n483 = local read "Gain Number"() -> (w227:i32[])
                      n484 = local read "GAIN"() -> (w223:u16)
                      n485 = local read "ADC Number"() -> (w228:i32[])
                      n486 = local read "ADC"() -> (w224:u16)
                      n487 = Index Array(array=w227, index=w223) -> (element=w225:i32)
                      n488 = Index Array(array=w228, index=w224) -> (element=w226:i32)
                      n489 = local read "Number of Areas :"() -> (w230:u16)
                      n490 = local read "areas :"() -> (w231:i32[][])
                      n491 = call "Setup CCD.vi"("numAreas"=w230, "areas :"=w231, "JYCCDLib.IJYCCDReqd"=w222, "entrée d'erreur (pas d'erreur)"=w234, "Acquisition type"=w232, "Gain"=w225, "Select ADC"=w226, "Integration time(ms)"="Integration time (ms) :") -> ("DataSize"=→"DataSize":i32)  [unwired: 1 out]
                      "JYCCDLib.IJYCCDReqd" <- w222
                    }
                    frame #2 {
                      w235 = TRUE ("Visible")
                      n492 = property on="Continuous" class="Bool (严格)"("Visible"=w235) -> ()  [unwired: 2 in, 2 out]
                      n493 = property on="Acquire" class="Bool"("Visible"=w235) -> ()  [unwired: 2 in, 2 out]
                      n494 = local write "indicator"("Ready !" ("indicator")) -> ()
                    }
                  }
                }
              }
              n495 = case shown="假" "Temperature" {
                tunnel: w95 -> [_ w209]
                tunnel: w94 -> [_ w208]
                frame False {
                  n496 = property on="temp graph" class="WFChart (严格)"("Visible"=FALSE) -> ()  [unwired: 2 in, 2 out]
                }
                frame True {
                  n497 = stacked-sequence {
                    tunnel: w209 -> [_ w214]
                    tunnel: w208 -> [_ w213]
                    frame #0 {
                      n498 = property on="temp graph" class="WFChart (严格)"("Visible"=TRUE) -> ()  [unwired: 2 in, 2 out]
                    }
                    frame #1 {
                      w212 = u16 0 items=["° Celsius", "Kelvin", "° Farenheit"] ("units")
                      n499 = call "read temperature.vi"("entrée d'erreur (pas d'erreur)"=w213, "units"=w212, "JYCCDLib.IJYCCDReqd"=w214) -> ("Current Temperature"=w211:dbl)
                      n500 = local write "temp graph"(w211) -> ()
                    }
                  }
                }
              }
              n501 = Wait Until Next ms Multiple(millisecond multiple=u32 50 ("n millisecondes")) -> ()  [unwired: 1 out]
            }
          }
          frame #7 {
            n502 = Close Reference(reference=w238, error in (no error)=w237) -> ()  [unwired: 1 out]
          }
        }
        n503 = stacked-sequence {
          seq-local: [_ _ w248 _ _] -> [_ _ _ w258 w263]
          seq-local: [_ _ w247 _ _] -> [_ _ _ w257 _]
          seq-local: [_ _ _ w256 _] -> [_ _ _ _ _]
          frame #0 {
            n504 = call "Get Monos From Config Browser.vi"() -> ("UniqueIDs"=w243:string[], "Mono ID"=w244:string[])  [unwired: 3 in, 1 out]
            n505 = Build Cluster Array(w244, w243) -> (w241:cluster{"String":string, "String":string}[])
            n506 = property on="Mono ID" class="CmbBox"("Strings And Values []"=w241) -> ()  [unwired: 2 in, 2 out]
            n507 = Index Array(array=w241, index=0) -> (element=w242:cluster{"String":string, "String":string})
            n508 = Unbundle(w242) -> ("String"=w239:string)  [unwired: 1 out]
            "Current UniqueID" <- w239
            n509 = local write "Mono ID"(w239) -> ()
          }
          frame #1 {
            n510 = while {
              stop <- "Connect" stop-if-true
              n511 = local read "Mono ID"() -> (w245:string)
              n512 = local write "Current UniqueID"(w245) -> ()
            }
          }
          frame #2 {
            n513 = local read "Mono ID"() -> (w250:string)
            n514 = call "JYInitMono.vi"("Unique ID"=w250, "Force Init"="Force\nInitialization") -> ("Refnum out"=w248:refnum<k7>, "Initialized"=→"Initialized JY":bool, "error out"=w247:errorcluster)  [unwired: 9 in, 2 out]
          }
          frame #3 {
            n515 = call "Show Current Grating.vi"("Refnum in"=w258, "error in (no error)"=w257) -> ("Gratings"=w259:dbl[], "Grating Index"=w253:i32, "Current Grating"=w255:dbl, "Current Description"=w252:string, "error out"=w256:errorcluster)  [unwired: 5 in, 4 out]
            "Gratings" <- w259
            n516 = local write "Current Grating"(w255) -> ()
            n517 = local write "Current Description"(w252) -> ()
            n518 = Number To Decimal String(number=w259) -> (decimal integer string=w261:string[])  [unwired: 1 in]
            n519 = Number To Decimal String(number=w253) -> (decimal integer string=w254:string)  [unwired: 1 in]
            n520 = property on="Target Grating" class="CmbBox"("Value"=w254) -> ()  [unwired: 2 in, 2 out]
            n521 = Build Cluster Array(w261, string[] ["1", "2", "3"]) -> (w262:cluster{"Numeric":string, string}[])
            n522 = property on="Target Grating" class="CmbBox"("Strings And Values []"=w262) -> ()  [unwired: 2 in, 2 out]
          }
          frame #4 {
            n523 = while {
              tunnel: w263 -> [w265]
              stop <- w264 stop-if-true
              n524 = stacked-sequence {
                seq-local: [w269 _ _ _ _] -> [_ w276 w287 _ w295]
                seq-local: [w268 _ _ _ _] -> [_ w275 w286 _ _]
                seq-local: [_ w274 _ _ _] -> [_ _ _ _ _]
                seq-local: [_ w273 _ _ _] -> [_ _ _ _ _]
                seq-local: [_ _ w279 _ _] -> [_ _ _ _ _]
                seq-local: [_ _ w278 _ _] -> [_ _ _ w289 _]
                tunnel: w265 -> [w267 _ _ w290 _]
                frame #0 {
                  n525 = call "Show Current Grating.vi"("Refnum in"=w267) -> ("Grating Index"=→"Grating Index":i32, "Current Grating"=→"Current Grating":dbl, "Current Description"=→"Current Description":string, "error out"=w268:errorcluster, "JYMONOLib.IJYMonoReqd"=w269:refnum<k7>)  [unwired: 6 in, 4 out]
                }
                frame #1 {
                  n526 = call "JYGetCurrentWL.vi"("error in (no error)"=w275, "JYMONOLib.IJYMonoReqd"=w276) -> ("error out"=w273:errorcluster, "Units"=→"Units":string, "Current WL"=→"Current WL":dbl, "JYMONOLib.IJYMonoReqd 2"=w274:refnum<k7>)  [unwired: 6 in]
                }
                frame #2 {
                  w284 = u16 1 items=["Entrance", "Exit"] ("Mirror Number")
                  w285 = u16 0 items=["Entrance", "Exit"] ("Mirror Number")
                  n527 = call "JYGetMirrorPos.vi"("error in (no error)"=w286, "Mirror"=w285, "Refnum In"=w287) -> ("error out"=w282:errorcluster, "Current Mirror Position"=→"Entrance Mirror\nPosition":i32, "Refnum Out"=w283:refnum<k7>)  [unwired: 1 in]
                  n528 = call "JYGetMirrorPos.vi"("error in (no error)"=w282, "Mirror"=w284, "Refnum In"=w283) -> ("error out"=w278:errorcluster, "Current Mirror Position"=→"Exit Mirror\nPosition":i32, "Refnum Out"=w279:refnum<k7>)  [unwired: 1 in]
                }
                frame #3 {
                  w292 = u16 0 items=["Front Entrance", "Side Entrance", "Front Exit", "Side Exit", "First Intermediate", "Second Intermediate"] ("Slit")
                  n529 = call "JYGetSlits.vi"("MonoRefNum IN"=w290, "Slit"=w292, "error in (no error)"=w289) -> ("Units"=→"Units 2":string, "Slit Width"=→"Front Entrance":dbl, "error out"=→"error out":errorcluster)  [unwired: 13 in, 1 out]
                }
                frame #4 {
                  n530 = case shown="真" "Move To\nTarget Positions" {
                    tunnel: w295 -> [_ w296]
                    frame False {
                    }
                    frame True {
                      n531 = stacked-sequence {
                        seq-local: [w298 _ _ _] -> [_ w304 _ _]
                        seq-local: [_ w302 _ _] -> [_ _ w319 _]
                        seq-local: [_ _ w306 _] -> [_ _ _ w325]
                        seq-local: [_ _ _ w322] -> [_ _ _ _]
                        tunnel: w296 -> [w300 w303 w317 w326]
                        frame #0 {
                          n532 = property on="Target Grating" class="CmbBox"() -> ("Value"=w297:string)  [unwired: 2 in, 2 out]
                          n533 = local read "error out"() -> (w299:errorcluster)
                          n534 = Decimal String To Number(string=w297) -> (number=w301:i32)  [unwired: 2 in, 1 out]
                          n535 = call "JYTurret.vi"("error in (no error)"=w299, "Grating Index"=w301, "JYMONOLib.IJYMonoReqd"=w300) -> ("error out"=w298:errorcluster)  [unwired: 2 out]
                        }
                        frame #1 {
                          # "Move Grating to Target Position"
                          n536 = call "JYMoveToWavelength.vi"("error in (no error)"=w304, "Target WL"="Target WL", "RefNum In"=w303) -> ("error out"=w302:errorcluster)  [unwired: 1 in, 2 out]
                        }
                        frame #2 {
                          w312 = u16 1 items=["Entrance", "Exit"] ("Mirror Number")
                          w311 = u16 0 items=["Entrance", "Exit"] ("Mirror Number")
                          w318 = u16 1 items=["Entrance", "Exit", "Front", "Side"] ("Mirror Number")
                          w321 = u16 0 items=["Entrance", "Exit", "Front", "Side"] ("Mirror Number")
                          # "Move Mirrors"
                          n537 = call "JYMirrorMove.vi"("error in (no error)"=w319, "Mirror Position"="Entrance Mirror", "Mirror Number"=w321, "RefNum In"=w317) -> ("error out"=w316:errorcluster)  [unwired: 6 in, 1 out]
                          n538 = call "JYMirrorMove.vi"("error in (no error)"=w316, "Mirror Position"="Exit Mirror", "Mirror Number"=w318, "RefNum In"=w317) -> ("error out"=w309:errorcluster, "MonoRefNum Out"=w310:refnum<k7>)  [unwired: 6 in]
                          n539 = call "JYGetMirrorPos.vi"("error in (no error)"=w309, "Mirror"=w311, "Refnum In"=w310) -> ("error out"=w314:errorcluster, "Current Mirror Position"=w308:i32, "Refnum Out"=w313:refnum<k7>)  [unwired: 1 in]
                          n540 = local write "Entrance Mirror\nPosition"(w308) -> ()
                          n541 = call "JYGetMirrorPos.vi"("error in (no error)"=w314, "Mirror"=w312, "Refnum In"=w313) -> ("error out"=w306:errorcluster, "Current Mirror Position"=w307:i32)  [unwired: 1 in, 1 out]
                          n542 = local write "Exit Mirror\nPosition"(w307) -> ()
                        }
                        frame #3 {
                          w324 = u16 0 items=["Front Entrance", "Side Entrance", "Front Exit", "Side Exit", "First Intermediate", "Second Intermediate"] ("Slit")
                          # "Set New Slit Positions"
                          n543 = call "JYSlits.vi"("JYMONOLib.IJYMonoReqd"=w326, "Slit"=w324, "error in (no error)"=w325, "Slit Width"="Target\nFront Entrance") -> ("error out"=w322:errorcluster)  [unwired: 1 in, 1 out]
                        }
                      }
                    }
                  }
                }
              }
              n544 = local read "Close"() -> (w264:bool)
            }
          }
        }
      }
    }
    n545 = event shown="[1] \"照明光\": 值改变" {
      selector: _ -> [_ _]
      dyn-events: _ -> [_ _]
      timeout: 0 -> [_ _]
      tunnel: "照明光" -> [_ w364]
      event Timeout {
        n546 = event-data() -> ()  [unwired: 1 in, 3 out]
      }
      event "照明光": Value Change {
        n547 = event-data() -> ()  [unwired: 1 in, 6 out]
        n548 = local read "stop bits (10: 1 bit)"() -> (w377:u16)
        n549 = local read "parity (0:none)"() -> (w376:enum16{"None", "Odd", "Even", "Mark", "Space"})
        n550 = local read "照明光VISA"() -> (w373:refnum<visa-resource-name>)
        n551 = local read "baud rate"() -> (w374:u32)
        n552 = local read "data bits (8)"() -> (w375:u16)
        n553 = call-poly "VISA Configure Serial Port"("VISA resource name"=w373, "baud rate (9600)"=w374, "data bits (8)"=w375, "parity (0:none)"=w376, "stop bits (10: 1 bit)"=w377) -> ("VISA resource name out"=w370:refnum<visa-resource-name>, "error out"=w369:errorcluster)  [unwired: 9 in]
        n554 = call <vilib>:"Simple Error Handler.vi"("error in (no error)"=w369) -> ()  [unwired: 4 in, 5 out]
        n555 = VISA Open(access mode=0, error in (no error)=w369, VISA resource name=w370) -> (VISA resource name=w372:refnum<visa-resource-name>, error out=w371:errorcluster)  [unwired: 2 in]
        n556 = stacked-sequence {
          tunnel: w372 -> [w382]
          tunnel: w371 -> [w381]
          tunnel: [w380] -> w367
          tunnel: [w379] -> w368
          tunnel: w364 -> [w378]
          frame #0 {
            n557 = case shown="假" w378 {
              tunnel: w382 -> [w388 w398]
              tunnel: [w386 w397] -> w380
              tunnel: w381 -> [w387 w396]
              tunnel: [w385 w395] -> w379
              frame False {
                n558 = Concatenate Strings(" \u0001\u0001¢", "\r") -> (w389:string)
                n559 = VISA Write(VISA resource name=w388, write buffer=w389, error in (no error)=w387) -> (VISA resource name out=w386:refnum<visa-resource-name>, error out=w385:errorcluster)  [unwired: 1 out]
                n560 = Wait (ms)(milliseconds to wait=50) -> ()  [unwired: 1 out]
              }
              frame True {
                w391 = " \u0001\u0000¡"  # Channel
                n561 = Wait (ms)(milliseconds to wait=50) -> ()  [unwired: 1 out]
                n562 = Concatenate Strings(w391, "\r") -> (w392:string)
                n563 = VISA Write(VISA resource name=w398, write buffer=w392, error in (no error)=w396) -> (VISA resource name out=w397:refnum<visa-resource-name>, error out=w395:errorcluster)  [unwired: 1 out]
              }
            }
          }
        }
        n564 = VISA Close(VISA resource name=w367, error in (no error)=w368) -> (error out=w366:errorcluster)
        n565 = call <vilib>:"Simple Error Handler.vi"("error in (no error)"=w366) -> ()  [unwired: 4 in, 5 out]
      }
    }
  }
